vi "Plot AS Effects by Wavelength.vi"() -> ()   [LabVIEW 2019]
uses:
  <vilib>/Analysis/baseanly.llb/Mean (DBL).vi
  <vilib>/Analysis/NI_AALBase.lvlib
panel:
  in  "Color 3":u32(colorbox)=16711680
  out "New Vector - Depth":dbl[](graph)
  out "Vector - Wavelength":dbl[](graph)
  out "Vector - Abs":dbl[](graph)
  out "Vector - Scattering":dbl[](graph)
  out "Vector - Depth":dbl[](graph)
  in  "Color 1":u32(colorbox)
  in  "Color 2":u32(colorbox)=16711680
  out "WD":dbl
  in  "Array 2":T1(array[cluster])
  out "Effects by Wavelength 2":cluster{dbl[], dbl[]}[](graph)
  out "Effects by Wavelength":cluster{dbl[], dbl[]}[](graph)
  out "Graphs":T2(array[cluster])
  out "Values":dbl[][][](array[numeric])
  out "Axis Vectors":T3
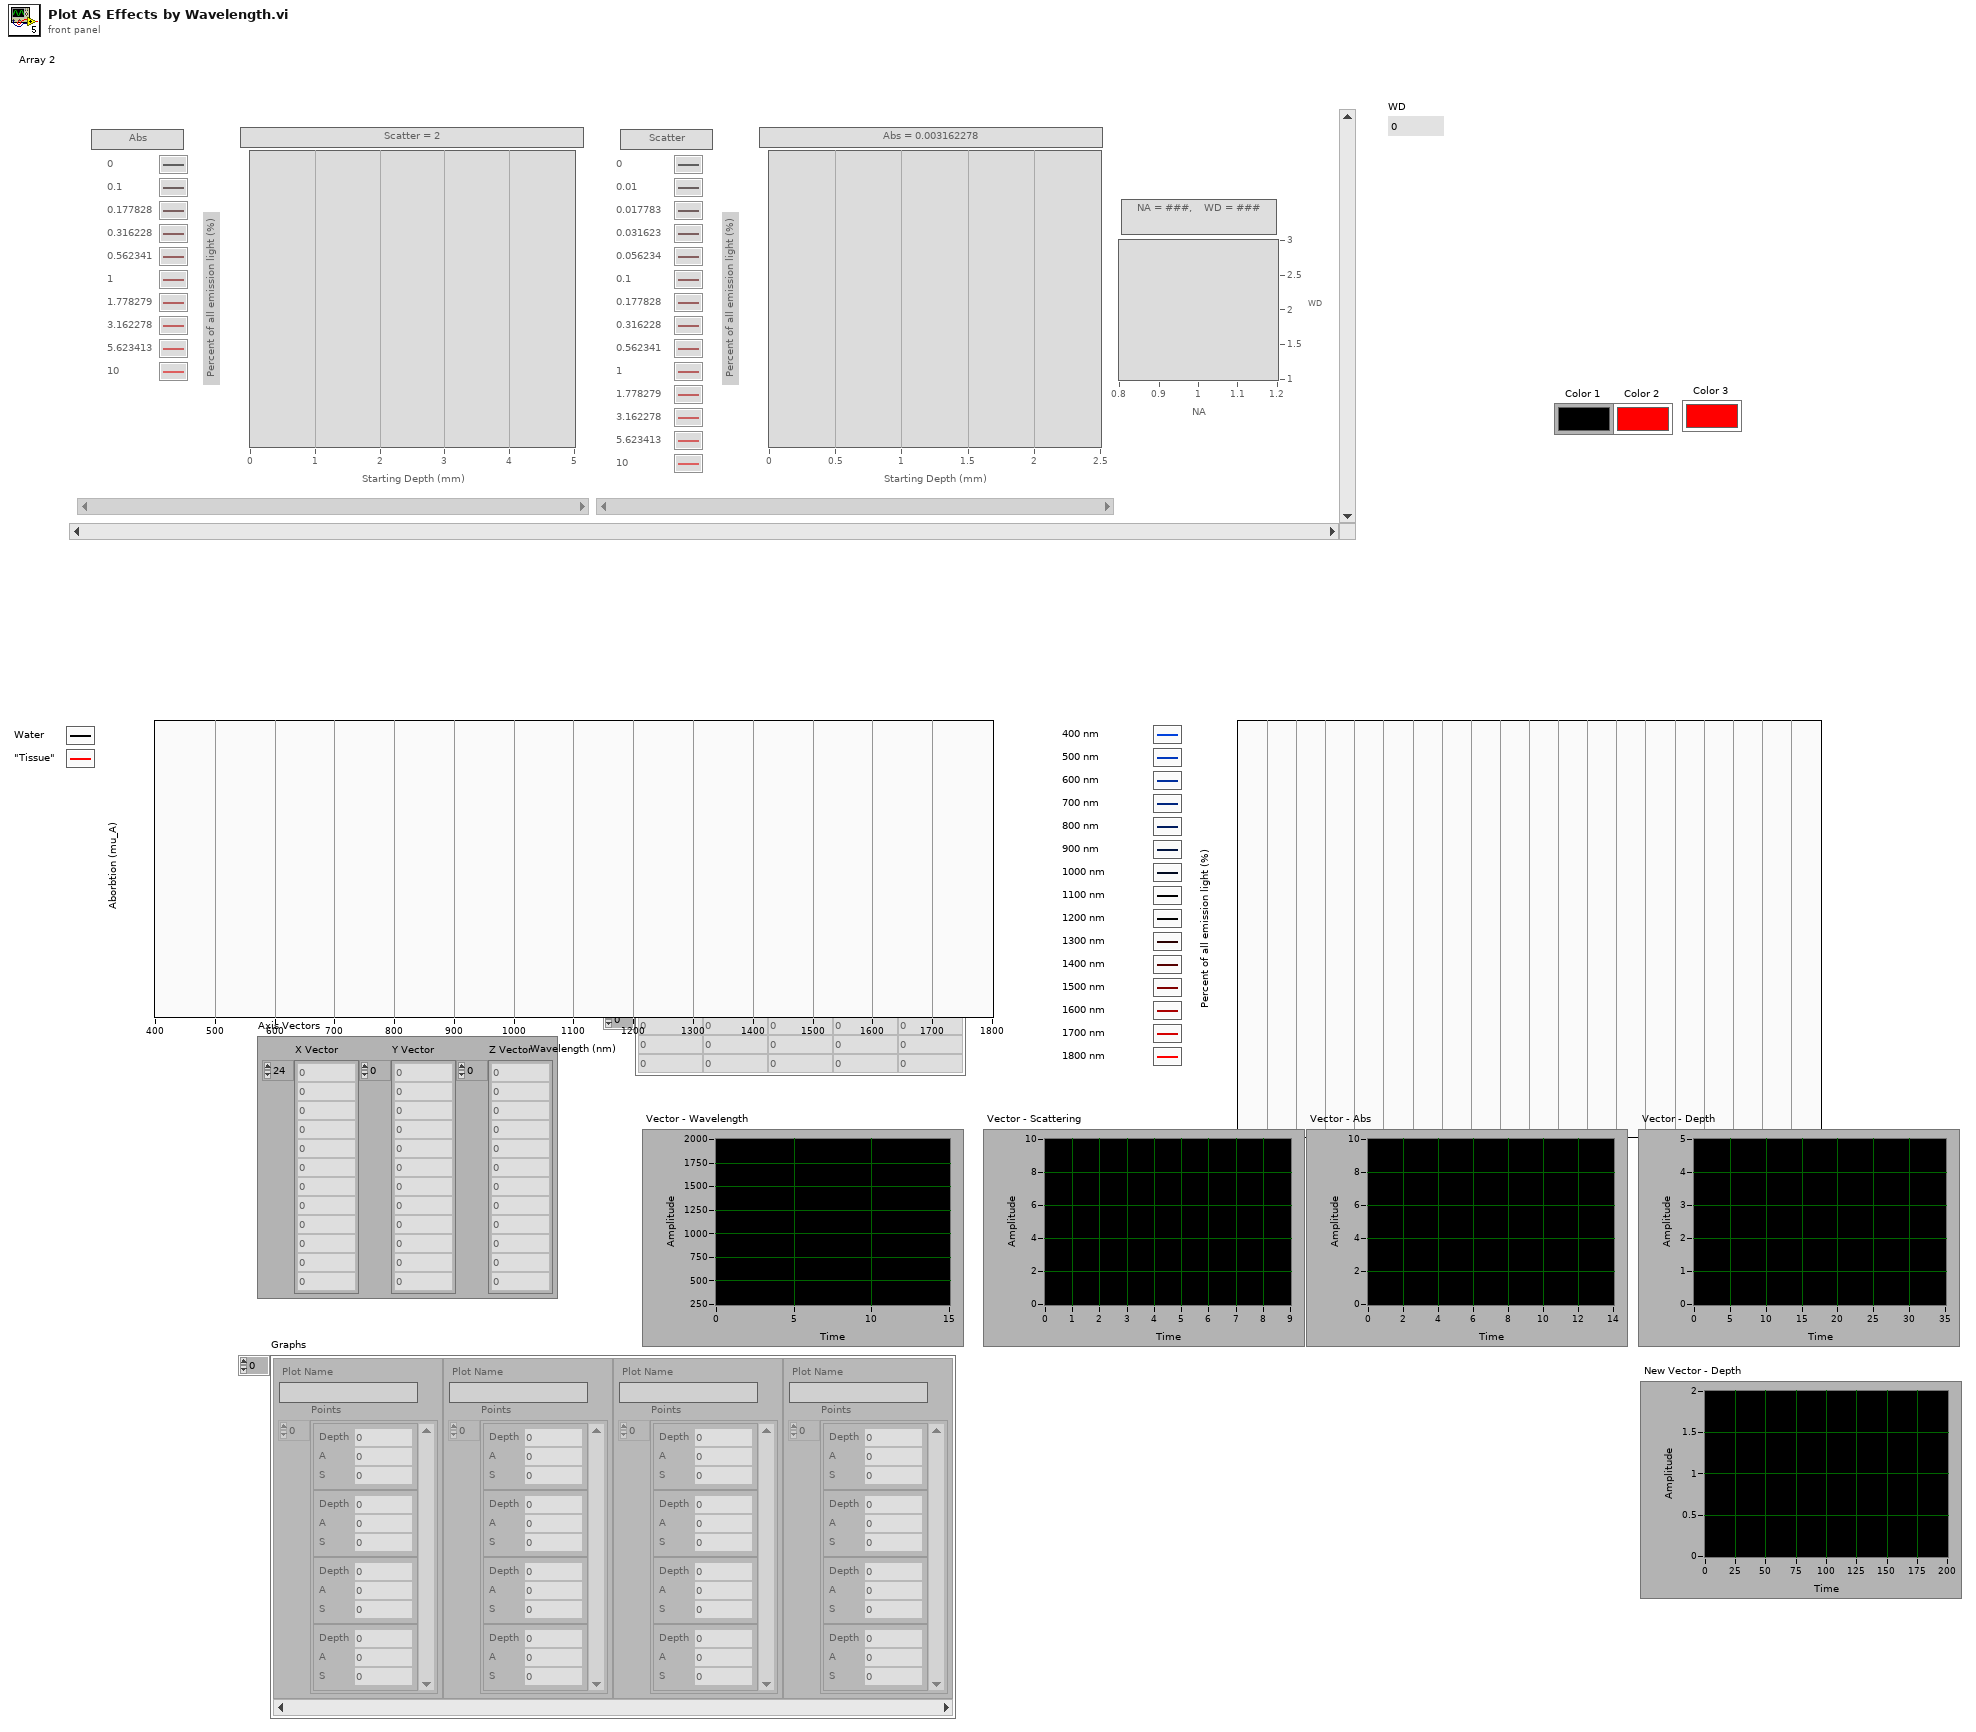
[diagram p1: front panel]
types:
  T1 = cluster{"Slab C=A, T=S 2":cluster{"Color and Time Graph":cluster{dbl[], dbl[]}[], "String":string, "String 2":string}[], "Slab C=S, T=A":cluster{"Color and Time Flipped Graph":cluster{dbl[], dbl[]}[], "String":string, "String 2":string}[], "Supra-Space Label":string, "Supra-Space Mini Map":cluster{dbl[], dbl[]}[]}[][]
  T2 = cluster{"Plot Name":string, "Points":cluster{"Depth":dbl, "A":dbl, "S":dbl}[]}[]
  T3 = cluster{"X Vector":dbl[], "Y Vector":dbl[], "Z Vector":dbl[]}
  T4 = cluster{"Slab C=A, T=S 2":cluster{"Color and Time Graph":cluster{dbl[], dbl[]}[], "String":string, "String 2":string}[], "Slab C=S, T=A":cluster{"Color and Time Flipped Graph":cluster{dbl[], dbl[]}[], "String":string, "String 2":string}[], "Supra-Space Label":string, "Supra-Space Mini Map":cluster{dbl[], dbl[]}[]}
  T5 = cluster{"Color and Time Graph":cluster{dbl[], dbl[]}[], "String":string, "String 2":string}[]
  T6 = cluster{string, cluster{dbl, "mean":dbl, "mean":dbl}[]}
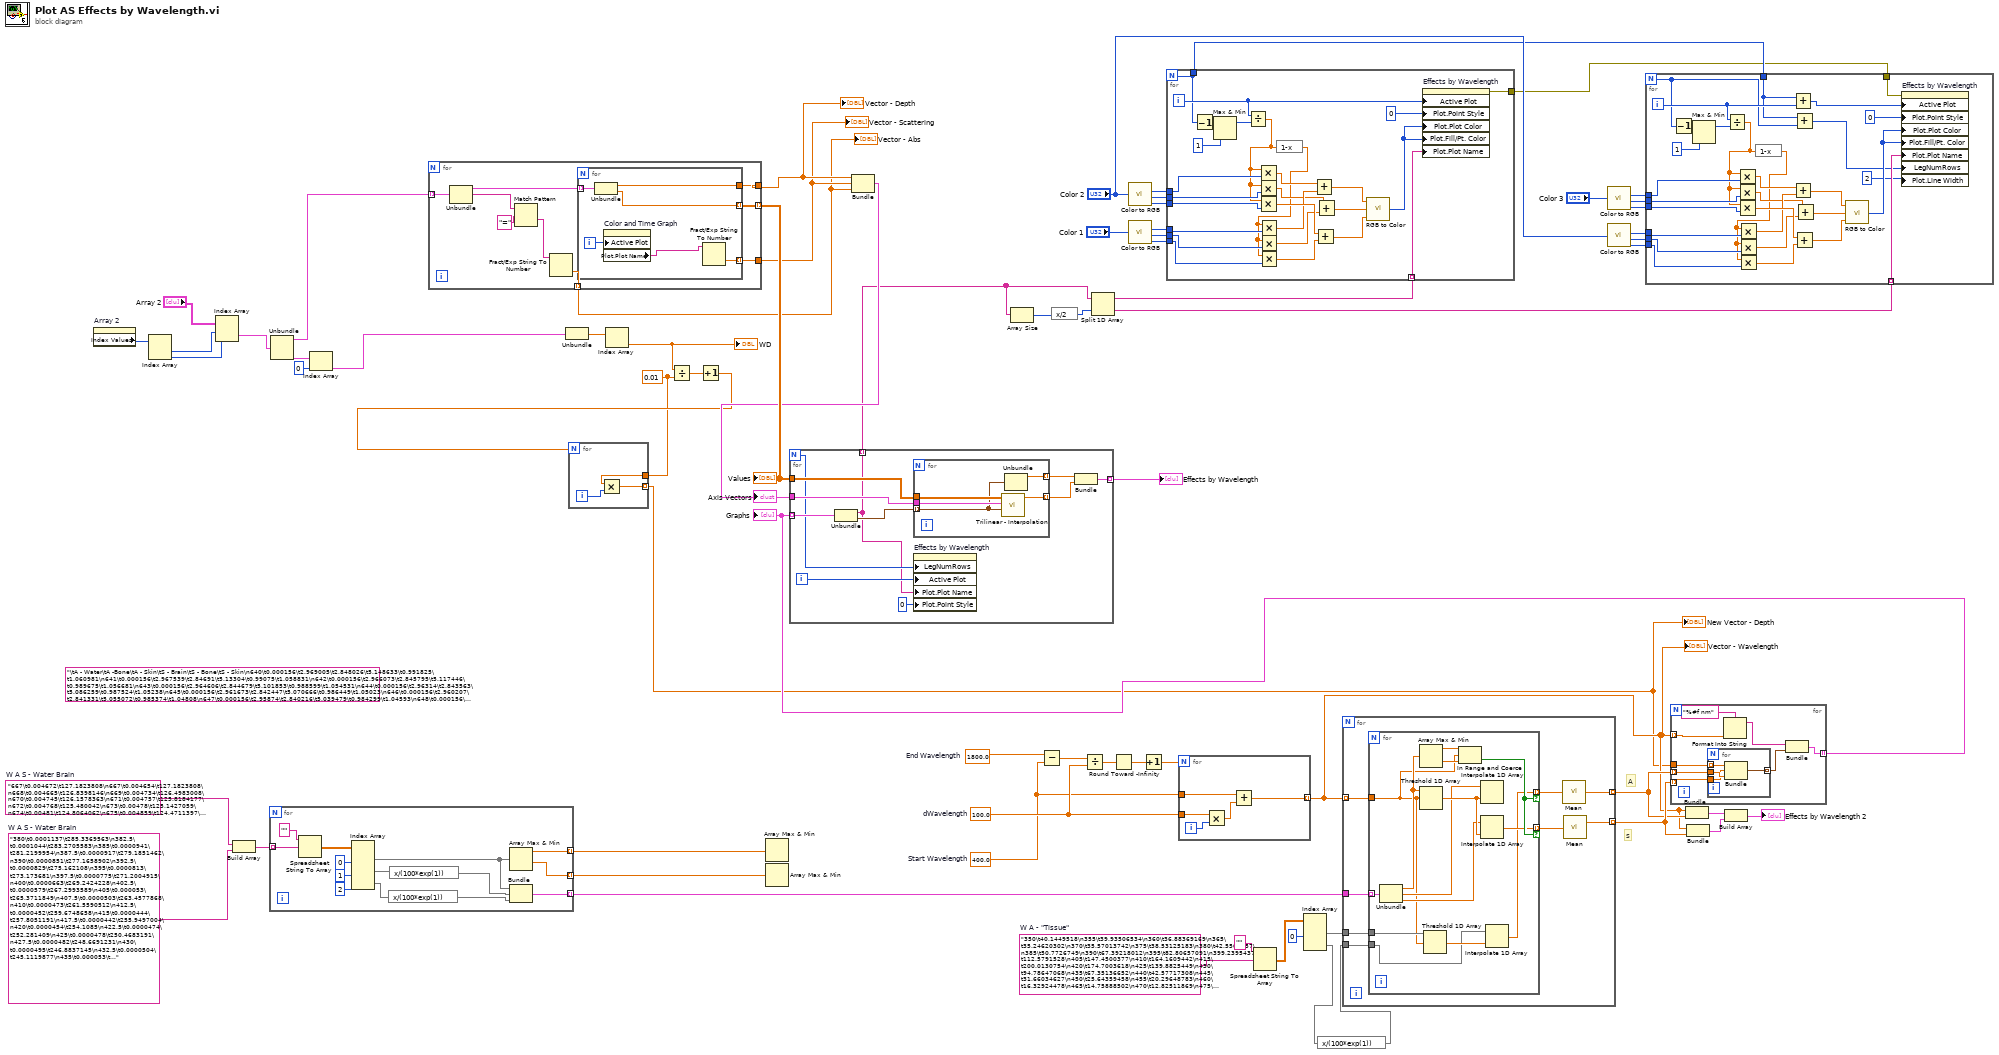
[diagram p0: block diagram]
diagram:
  w6 = "350\t40.1449518\n355\t39.93506534\n360\t36.88369169\n365\t35.24620302\n370\t35.57013742\n375\t38.53125183\n380\t42.5502257\n385\t50.7726749\n390\t67.39218012\n395\t82.80657091\n399.2395437\t112.5791528\n405\t147.4500377\n410\t164.1609442\n415\t200.0130754\n420\t174.7003618\n425\t139.8825449\n430\t94.78647068\n435\t67.35136652\n440\t42.57717308\n445\t31.66034627\n450\t25.64359458\n455\t20.29648783\n460\t16.32924478\n465\t14.75888502\n470\t12.82511869\n475\t11.17993961\n480\t10.46687393\n485\t9.635143522\n490\t9.070944487\n495\t8.526317886\n500\t7.944068527\n505\t7.865547206\n510\t7.700269633\n515\t8.291297449\n520\t10.14066835\n525\t11.9882333\n530\t15.26433309\n535\t18.44669386\n540\t20.06695237\n545\t18.73208821\n550\t16.22399299\n555\t14.2878093\n560\t12.8688612\n565\t14.58935325\n570\t17.42869783\n575\t20.36742691\n580\t18.23646398\n585\t10.31152261\n590\t5.804468682\n595\t3.200359382\n595.4372624\t2.526479178\n600\t1.325426446\n600\t1.770203167\n605\t0.905448403\n610\t0.676965894\n615\t0.503195306\n620\t0.392170144\n625\t0.332756249\n630\t0.262305095\n634.9809886\t0.217724537\n645\t0.185248241\n650\t0.170446221\n655\t0.160044101\n660\t0.149831499\n665\t0.141595627\n670\t0.138511159\n675\t0.129196263\n680\t0.125722595\n690\t0.126946584\n695\t0.124976166\n700\t0.129381074\n705\t0.132661431\n710\t0.139652936\n715\t0.14352338\n720\t0.152435705\n725\t0.161474142\n730\t0.171771141\n735\t0.18862398\n745\t0.221099782\n750\t0.22825934\n755\t0.244064738\n760\t0.256883178\n765\t0.263882999\n770\t0.280363387\n775\t0.286602175\n780\t0.295060702\n785\t0.303809506\n790\t0.307356933\n795\t0.318984637\n800\t0.318026227\n805\t0.338556011\n810\t0.34704747\n815\t0.356807245\n820\t0.375667111\n825\t0.384516469\n830\t0.398029786\n835\t0.396401541\n840\t0.417394879\n845\t0.429067561\n850\t0.437298168\n855\t0.446551299\n860\t0.451377547\n865\t0.463879395\n870\t0.470866705\n875\t0.481680183\n880\t0.491192221\n885\t0.489926302\n890\t0.501477925\n895\t0.49950668\n900\t0.510710562\n905\t0.519552579\n910\t0.524750128\n915\t0.530537466\n925\t0.573360204\n930\t0.60325251\n935\t0.652823151\n940\t0.692541\n945\t0.720914259\n950\t0.750743305\n955\t0.763756172\n960\t0.780625173\n965\t0.778987403\n970\t0.77900704\n975\t0.779424043\n980\t0.747885452\n985\t0.73604543\n990\t0.726568849\n995\t0.703054919\n1005\t0.640459172\n1010\t0.631019981\n1015\t0.605494507\n1020\t0.593542803\n1025\t0.577902355\n1030\t0.551214031\n1035\t0.52392221\n1040\t0.518082861\n1045\t0.500688926\n1050\t0.494941961\n1055\t0.490235149\n1060\t0.48120179\n1065\t0.481679295\n1070\t0.48195256\n1075\t0.485853895\n1080\t0.4910582\n1085\t0.497427334\n1090\t0.50207148\n1095\t0.508977606\n1100\t0.532046234\n1105\t0.600127102\n1110\t0.673697238\n1115\t0.737622627\n1120\t0.772759251\n1125\t0.814359969\n1130\t0.838194475\n1135\t0.869665233\n1140\t0.907133059\n1145\t0.953829503\n1150\t1.003180636\n1155\t1.029832409\n1160\t1.083120174\n1165\t1.096412814\n1170\t1.130980203\n1175\t1.166048877\n1180\t1.203815485\n1185\t1.212393847\n1190\t1.211334263\n1195\t1.202370275\n1205\t1.147063957\n1210\t1.14480334\n1215\t1.133019682\n1220\t1.123946852\n1225\t1.106075064\n1230\t1.096576616\n1235\t1.079514875\n1240\t1.071173164\n1245\t1.059883956\n1250\t1.072363897\n1255\t1.0802166\n1260\t1.078551226\n1265\t1.103983447\n1270\t1.100520936\n1275\t1.135796167\n1280\t1.14528267\n1285\t1.167016028\n1290\t1.195557654\n1295\t1.212261598\n1300\t1.2528459\n1305\t1.308400792\n1310\t1.364621761\n1315\t1.389609815\n1320\t1.4575677\n1325\t1.575745643\n1330\t1.642634392\n1335\t1.755508464\n1340\t1.848687825\n1345\t2.029670114\n1350\t2.17465122\n1355\t2.387127826\n1360\t2.725223028\n1365\t3.099532802\n1370\t3.821496699\n1375\t4.648516526\n1380\t5.387499682\n1385\t6.405116468\n1390\t7.584722337\n1395\t9.418840656\n1400\t11.03777779\n1405\t13.21466549\n1410\t13.69427731\n1415\t15.97982135\n1420\t17.72345799\n1425\t19.17000525\n1430\t20.47042995\n1435\t21.66822653\n1440\t22.35531618\n1445\t22.54541213\n1450\t22.54017823\n1455\t22.49699476\n1460\t21.75668848\n1465\t20.74741653\n1470\t19.36922072\n1475\t17.65023139\n1480\t16.86251361\n1485\t16.06846979\n1490\t15.26443185\n1495\t14.62214346\n1500\t13.84442241\n1505\t13.18146958\n1510\t12.67839918\n1515\t11.9108062\n1520\t11.18185614\n1525\t10.75134473\n1530\t10.4644584\n1535\t9.960937877\n1540\t9.500840415\n1545\t9.043900037\n1550\t8.59139503\n1555\t8.246474109\n1560\t7.787345858\n1565\t7.426642643\n1570\t7.139772584\n1575\t6.843935199\n1580\t6.471933806\n1585\t6.319686367\n1590\t5.977637406\n1595\t5.598292552\n1605\t5.088303625\n1610\t5.218338934\n1615\t5.040110752\n1620\t4.814515468\n1625\t4.683044053\n1630\t4.549824308\n1635\t4.321414117\n1640\t4.234176712\n1645\t4.146068224\n1650\t3.980268622\n1655\t3.983481534\n1660\t3.85388727\n1665\t3.845634415\n1670\t3.844005614\n1675\t3.844025551\n1680\t3.844058246\n1685\t3.843825774\n1690\t3.842531257\n1695\t3.853006003\n1700\t3.812756788\n1705\t3.993046892\n1710\t4.118971368\n1715\t4.251713554\n1720\t4.391401881\n1725\t4.600454261\n1730\t4.81775904\n1735\t5.023875653\n1740\t5.129042685\n1745\t5.3305322\n1750\t5.565698916\n1755\t5.723454663\n1760\t5.899438259\n1765\t6.09319314\n1770\t6.192110419\n1775\t6.463619324\n1780\t6.595917836\n1785\t6.588767301\n1790\t6.565100324\n1795\t6.375994569\n1805\t6.467197127\n1810\t6.978660754\n1815\t7.113147564\n1820\t7.275532454\n1825\t7.634295763\n1830\t7.706014548\n1835\t8.113183192\n1840\t8.510845753\n1845\t9.371650726\n1850\t10.0057303\n1855\t10.67490914\n1860\t12.92043247\n1865\t14.73406603\n1870\t18.52749241\n1875\t22.06098103\n1880\t26.11212325\n1885\t33.31211384\n1890\t38.47333909\n1895\t44.54571665\n1900\t54.57154096\n1905\t61.23449331\n1910\t72.21092231\n1915\t81.43598948\n1920\t88.57123236\n1925\t90.28969599\n1930\t89.89725373\n1935\t91.92493944\n1940\t91.7611798\n1945\t88.90434479\n1950\t86.04389\n1955\t83.52977617\n1960\t79.95489241\n1965\t78.8923421\n1970\t76.59635098\n1975\t72.69370288\n1985.551331\t62.41825263\n1996.197719\t53.86107465"  # W A - "Tissue"
  w24 = 1800.0  # End Wavelength
  w31 = 400.0  # Start Wavelength
  w66 = 100.0  # dWavelength
  w40 = 0.01 ("y")
  w61 = "667\t0.004672\t127.1823808\n667\t0.004654\t127.1823808\n668\t0.004665\t126.8398146\n669\t0.004734\t126.4983008\n670\t0.004745\t126.1578363\n671\t0.004757\t125.8184177\n672\t0.004768\t125.480042\n673\t0.00478\t125.1427059\n674\t0.00481\t124.8064062\n675\t0.004859\t124.4711397\n676\t0.004908\t124.1369033\n676\t0.004852\t124.1369033\n677\t0.0049\t123.8036937\n678\t0.00493\t123.4715078\n679\t0.004978\t123.1403426\n680\t0.005008\t122.8101948\n681\t0.005038\t122.4810613\n682\t0.00503\t122.152939\n683\t0.005078\t121.8258247\n684\t0.005126\t121.4997155\n685\t0.005173\t121.1746082\n686\t0.005202\t120.8504998\n687\t0.00525\t120.5273871\n688\t0.005315\t120.2052671\n689\t0.005362\t119.8841368\n689.7\t0.00543\t119.6599327\n690\t0.005536\t119.563993\n691\t0.005638\t119.2448329\n692\t0.00572\t118.9266533\n693\t0.005803\t118.6094513\n694\t0.005921\t118.2932238\n695\t0.006021\t117.9779679\n696\t0.006139\t117.6636805\n697\t0.006256\t117.3503587\n698\t0.006391\t117.0379995\n699\t0.006526\t116.7266001\n700\t0.006678\t116.4161573\n701\t0.00683\t116.1066683\n702\t0.006981\t115.7981301\n703\t0.00715\t115.4905399\n704\t0.007354\t115.1838947\n705\t0.007522\t114.8781916\n706\t0.007725\t114.5734278\n707\t0.007927\t114.2696002\n708\t0.008147\t113.9667061\n709\t0.008401\t113.6647426\n710\t0.008655\t113.3637068\n711\t0.008979\t113.0635959\n712\t0.009301\t112.7644071\n713\t0.009694\t112.4661374\n714\t0.010067\t112.1687841\n715\t0.010492\t111.8723444\n716\t0.010952\t111.5768154\n717\t0.01141\t111.2821944\n718\t0.011901\t110.9884786\n719\t0.012427\t110.6956652\n721\t0.01295\t110.1127344\n722\t0.013489\t109.8226115\n723\t0.014061\t109.5333799\n724\t0.014667\t109.245037\n725\t0.015253\t108.95758\n726\t0.015924\t108.6710061\n727\t0.016646\t108.3853127\n728\t0.017607\t108.100497\n729\t0.018444\t107.8165563\n730\t0.019624\t107.533488\n731\t0.020801\t107.2512894\n732\t0.021974\t106.9699578\n733\t0.023144\t106.6894905\n734\t0.024482\t106.4098849\n735\t0.025304\t106.1311383\n736\t0.026123\t105.8532482\n738\t0.026733\t105.3000265\n739\t0.027377\t105.0246898\n740\t0.02768\t104.750199\n741\t0.027982\t104.4765515\n742\t0.028113\t104.2037448\n743\t0.028245\t103.9317762\n744\t0.028376\t103.6606432\n745\t0.028338\t103.3903432\n746\t0.028468\t103.1208736\n747\t0.02843\t102.8522319\n748\t0.02856\t102.5844156\n750\t0.028484\t102.0512489\n751\t0.028613\t101.7858934\n752\t0.028575\t101.5213533\n753\t0.028704\t101.2576258\n754\t0.028666\t100.9947086\n755\t0.028794\t100.7325992\n756\t0.028756\t100.4712951\n758\t0.028681\t99.95109276\n759\t0.028643\t99.69218966\n760\t0.028605\t99.43408199\n761\t0.028733\t99.1767673\n762\t0.028695\t98.92024318\n763\t0.028657\t98.66450717\n765\t0.028582\t98.15538985\n766\t0.028545\t97.90200372\n767\t0.028344\t97.64939606\n768\t0.028307\t97.3975645\n769\t0.02827\t97.14650665\n770\t0.028234\t96.89622012\n772\t0.027998\t96.39795159\n773\t0.027799\t96.14996486\n774\t0.027763\t95.90274003\n775\t0.027565\t95.65627475\n776\t0.027529\t95.41056669\n778\t0.027297\t94.92141292\n779\t0.027101\t94.67796259\n780\t0.026905\t94.43526021\n781\t0.026549\t94.1933035\n783\t0.02632\t93.71161788\n784\t0.026127\t93.47188442\n785\t0.025933\t93.2328875\n786\t0.02558\t92.99462485\n787\t0.025229\t92.75709422\n789\t0.025005\t92.28422003\n790\t0.024656\t92.04887198\n791\t0.024465\t91.81424701\n792\t0.024117\t91.58034287\n794\t0.02374\t91.11468828\n795\t0.023552\t90.88293341\n796\t0.023365\t90.65189056\n797\t0.023178\t90.42155755\n799\t0.022805\t89.96301233\n800\t0.022462\t89.73479577\n801\t0.022434\t89.50728037\n803\t0.022222\t89.05434442\n804\t0.022038\t88.82891958\n805\t0.022011\t88.60418731\n807\t0.021956\t88.15679201\n808\t0.021773\t87.93412473\n809\t0.021902\t87.71214156\n810\t0.021875\t87.49084039\n812\t0.021976\t87.05027569\n813\t0.022103\t86.83100798\n814\t0.02223\t86.61241393\n816\t0.022484\t86.17723855\n817\t0.022764\t85.96065309\n818\t0.023043\t85.74473304\n820\t0.023294\t85.31488105\n821\t0.023878\t85.10094502\n822\t0.02446\t84.88766628\n824\t0.025163\t84.46307255\n825\t0.026199\t84.25175355\n826\t0.027689\t84.04108379\n828\t0.029139\t83.62168401\n829\t0.031075\t83.41295003\n831\t0.032966\t82.99740397\n832\t0.034588\t82.79058797\n833\t0.036055\t82.58440737\n835\t0.037022\t82.17394459\n836\t0.037879\t81.96965851\n838\t0.038539\t81.56296733\n839\t0.039092\t81.36055837\n840\t0.039494\t81.15877128\n842\t0.039997\t80.75705505\n843\t0.040397\t80.55712211\n845\t0.040748\t80.15909711\n846\t0.041145\t79.96100129\n848\t0.041493\t79.56663361\n849\t0.042036\t79.37035802\n850\t0.041986\t79.17468545\n851\t0.042232\t78.97961405\n853\t0.042723\t78.59126737\n855\t0.043064\t78.20530328\n856\t0.043601\t78.01321013\n858\t0.043792\t77.63079252\n859\t0.044326\t77.44046445\n861\t0.044661\t77.06156075\n862\t0.045047\t76.87298154\n864\t0.045524\t76.49755946\n865\t0.046052\t76.31071304\n866\t0.04658\t76.12444067\n868\t0.047052\t75.75361104\n870\t0.047521\t75.38505651\n871\t0.048332\t75.20162805\n873\t0.048941\t74.83646005\n874\t0.049604\t74.65471706\n876\t0.050495\t74.29290446\n877\t0.051154\t74.11283144\n879\t0.052038\t73.75434342\n880\t0.052979\t73.57592502\n882\t0.053856\t73.22073103\n883\t0.054649\t73.04395206\n885\t0.055661\t72.69202182\n887\t0.056527\t72.34225074\n888\t0.057454\t72.16817074\n890\t0.058314\t71.82161359\n891\t0.059235\t71.64913316\n893\t0.060088\t71.3057604\n895\t0.060936\t70.96449431\n896\t0.06185\t70.79464721\n898\t0.062692\t70.4565169\n899\t0.063601\t70.28823047\n901\t0.064575\t69.95320712\n902\t0.065618\t69.78646702\n904\t0.066724\t69.45452208\n906\t0.067686\t69.12461369\n907\t0.068997\t68.9604193\n909\t0.070366\t68.63354232\n911\t0.071867\t68.30867081\n912\t0.073579\t68.14698324\n914\t0.075618\t67.82509686\n916\t0.077922\t67.50518531\n917\t0.080852\t67.34596631\n919\t0.084095\t67.02899432\n921\t0.088006\t66.71396701\n922\t0.09268\t66.55717888\n924\t0.098192\t66.24504626\n926\t0.104222\t65.93482863\n928\t0.11131\t65.62651424\n929\t0.119441\t65.47306711\n931\t0.128093\t65.16758572\n933\t0.137382\t64.86397852\n935\t0.146496\t64.56223401\n936\t0.155737\t64.41205668\n938\t0.168802\t64.1130848\n940\t0.181811\t63.81594716\n941\t0.196308\t63.66806267\n943\t0.21055\t63.37365533\n945\t0.228721\t63.08105424\n947\t0.246816\t62.79024831\n949\t0.270131\t62.50122654\n950\t0.297625\t62.35738128\n952\t0.327359\t62.07101523\n954\t0.362238\t61.78640609\n956\t0.393028\t61.50354308\n958\t0.418442\t61.22241549\n960\t0.438514\t60.94301267\n961\t0.453749\t60.80395475\n963\t0.463246\t60.52711927\n965\t0.470099\t60.25198223\n967\t0.475625\t59.97853321\n969\t0.478534\t59.70676185\n971\t0.48143\t59.43665786\n973\t0.484315\t59.16821101\n974\t0.486399\t59.03460584\n976\t0.486689\t58.76862566\n978\t0.485694\t58.50427732\n980\t0.482138\t58.2415508\n982\t0.478597\t57.98043617\n984\t0.473793\t57.72092353\n986\t0.467734\t57.46300304\n988\t0.460428\t57.20666495\n990\t0.453151\t56.95189954\n992\t0.44337\t56.69869717\n994\t0.436157\t56.44704824\n996\t0.426449\t56.19694323\n998\t0.41678\t55.94837266\n1000\t0.40715\t55.70132712\n1002\t0.396305\t55.45579725\n1004\t0.386754\t55.21177376\n1006\t0.375992\t54.9692474\n1008\t0.364026\t54.72820898\n1010\t0.352107\t54.48864938\n1012\t0.340236\t54.25055952\n1014\t0.32965\t54.0139304\n1016\t0.319107\t53.77875304\n1018\t0.308604\t53.54501853\n1020\t0.295679\t53.31271804\n1022\t0.284034\t53.08184275\n1024\t0.272435\t52.85238393\n1026\t0.262106\t52.62433288\n1028\t0.250594\t52.39768097\n1030\t0.239127\t52.17241961\n1033\t0.229917\t51.83711621\n1035\t0.21976\t51.61529403\n1037\t0.210853\t51.39483277\n1039\t0.201981\t51.17572408\n1041\t0.19435\t50.95795966\n1043\t0.186749\t50.74153128\n1046\t0.179005\t50.41937583\n1048\t0.171469\t50.20625176\n1050\t0.166355\t49.99443524\n1052\t0.16126\t49.78391826\n1054\t0.156185\t49.57469285\n1057\t0.152176\t49.26325908\n1059\t0.149515\t49.05722801\n1061\t0.14568\t48.85246098\n1063\t0.144224\t48.64895024\n1066\t0.142639\t48.34602281\n1068\t0.141195\t48.14561916\n1070\t0.140931\t47.94644503\n1073\t0.140537\t47.64997268\n1075\t0.141445\t47.45383944\n1077\t0.143516\t47.25890951\n1080\t0.144281\t46.96875469\n1082\t0.147498\t46.77680085\n1084\t0.151863\t46.58602469\n1087\t0.156068\t46.30205278\n1089\t0.160397\t46.11418929\n1091\t0.165862\t45.92747837\n1094\t0.171151\t45.64955762\n1096\t0.177718\t45.46569731\n1098\t0.18655\t45.28296502\n1101\t0.19289\t45.01096649\n1103\t0.200515\t44.83102406\n1106\t0.207925\t44.56317826\n1108\t0.216622\t44.3859831\n1111\t0.225086\t44.12222664\n1113\t0.233714\t43.9477368\n1116\t0.235338\t43.68800723\n1118\t0.245033\t43.51618141\n1121\t0.257829\t43.26041726\n1123\t0.271917\t43.09121479\n1126\t0.289049\t42.83935551\n1128\t0.316387\t42.67273633\n1131\t0.353325\t42.42472231\n1133\t0.403721\t42.26064699\n1136\t0.471239\t42.01641952\n1139\t0.557157\t41.77443617\n1141\t0.651997\t41.61435048\n1144\t0.753543\t41.37606161\n1146\t0.859689\t41.21842002\n1149\t0.949313\t40.98376922\n1152\t1.040653\t40.75127455\n1154\t1.09983\t40.59746616\n1157\t1.140423\t40.36852109\n1160\t1.169972\t40.14167972\n1162\t1.189588\t39.99161131\n1165\t1.197311\t39.76823324\n1168\t1.204994\t39.54690771\n1171\t1.212639\t39.32761587\n1173\t1.231997\t39.1825419\n1176\t1.228854\t38.96659809\n1179\t1.236386\t38.75263852\n1182\t1.243879\t38.54064495\n1184\t1.252392\t38.4003992\n1187\t1.259813\t38.19164224\n1190\t1.267197\t37.98480347\n1193\t1.274544\t37.77986528\n1196\t1.281854\t37.57681019\n1199\t1.278646\t37.37562091\n1201\t1.266054\t37.24252281\n1204\t1.273336\t37.04440518\n1207\t1.25976\t36.84810799\n1210\t1.256637\t36.65361451\n1213\t1.243169\t36.46090816\n1216\t1.240102\t36.26997252\n1219\t1.216433\t36.08079133\n1222\t1.213447\t35.89334846\n1225\t1.200217\t35.70762794\n1228\t1.197284\t35.52361394\n1231\t1.184158\t35.34129078\n1234\t1.171096\t35.16064293\n1237\t1.158097\t34.981655\n1240\t1.155295\t34.80431172\n1243\t1.142397\t34.62859799\n1246\t1.129561\t34.45449883\n1250\t1.115894\t34.22485256\n1253\t1.103193\t34.05446328\n1256\t1.100558\t33.88563965\n1259\t1.097935\t33.71836729\n1262\t1.085368\t33.55263193\n1265\t1.082794\t33.38841946\n1269\t1.079381\t33.17181427\n1272\t1.086714\t33.011101\n1275\t1.103869\t32.85186448\n1278\t1.111111\t32.69409112\n1282\t1.137051\t32.48597947\n1285\t1.163734\t32.33156811\n1288\t1.180536\t32.17857559\n1292\t1.215787\t31.97677011\n1295\t1.251785\t31.8270377\n1298\t1.297299\t31.67868113\n1302\t1.351223\t31.48299074\n1305\t1.415522\t31.3377955\n1308\t1.489134\t31.19393441\n1312\t1.580374\t31.0041738\n1315\t1.672331\t30.86337825\n1319\t1.791113\t30.67766125\n1322\t1.910621\t30.53986591\n1326\t2.04701\t30.35810636\n1329\t2.203133\t30.2232473\n1333\t2.356784\t30.04536086\n1336\t2.539611\t29.91337552\n1340\t2.700832\t29.73927966\n1344\t2.889143\t29.56731348\n1347\t3.097279\t29.43972075\n1351\t3.236933\t29.27141899\n1355\t3.394311\t29.10517603\n1358\t3.553377\t28.98182973\n1362\t3.72747\t28.81912923\n1366\t3.955739\t28.65841902\n1369\t4.222447\t28.53917781\n1373\t4.640313\t28.38189217\n1377\t5.183514\t28.22653056\n1381\t5.987452\t28.07306945\n1385\t7.204114\t27.9214856\n1388\t8.781973\t27.80901582\n1392\t11.013629\t27.66066207\n1396\t13.952631\t27.51412309\n1400\t16.964599\t27.36937668\n1404\t19.690893\t27.22640092\n1408\t22.312447\t27.08517414\n1412\t24.652156\t26.94567496\n1416\t26.357429\t26.80788224\n1420\t27.699111\t26.6717751\n1424\t29.121504\t26.53733292\n1428\t30.271928\t26.40453534\n1432\t31.064909\t26.27336224\n1437\t32.006203\t26.11165004\n1440\t32.201323\t26.01581023\n1445\t32.524722\t25.8580302\n1449\t32.69511\t25.73354236\n1453\t32.778075\t25.61057735\n1457\t32.688087\t25.48911654\n1462\t32.404388\t25.33937779\n1466\t31.544503\t25.22123449\n1470\t30.603813\t25.10453641\n1474\t29.668228\t24.98926587\n1479\t28.208484\t24.84715859\n1484\t26.927936\t24.70722093\n1488\t25.75768\t24.59681064\n1492\t24.08835\t24.48775098\n1497\t22.916627\t24.35330057\n1501\t21.599757\t24.24721971\n1506\t20.443298\t24.1164416\n1510\t19.224049\t24.01325817\n1515\t18.082301\t23.88605207\n1519\t17.04195\t23.78568694\n1524\t16.079017\t23.66195527\n1529\t15.368942\t23.54011268\n1533\t14.591088\t23.44397934\n1538\t13.8083\t23.32546469\n1543\t12.786261\t23.20875946\n1548\t12.176715\t23.09383602\n1552\t11.659519\t23.00316187\n1557\t10.976405\t22.89137739\n1562\t10.458567\t22.78129958\n1567\t9.944032\t22.67290238\n1572\t9.51271\t22.56616013\n1577\t9.163808\t22.46104757\n1582\t8.817112\t22.35753981\n1587\t8.4726\t22.25561236\n1592\t8.130252\t22.15524108\n1597\t7.868735\t22.05640222\n1602\t7.608851\t21.95907237\n1607\t7.381863\t21.86322851\n1612\t7.19526\t21.76884795\n1618\t6.989946\t21.65749138\n1623\t6.805816\t21.5662519\n1628\t6.661411\t21.47640542\n1634\t6.49083\t21.37039848\n1640\t6.356022\t21.26633071\n1644\t6.267897\t21.19801197\n1650\t6.161329\t21.09709765\n1655\t6.051599\t21.01441397\n1661\t5.984346\t20.91685818\n1666\t5.921129\t20.83692631\n1672\t5.877333\t20.74261729\n1677\t5.83733\t20.66534563\n1683\t5.838919\t20.57417532\n1689\t5.833057\t20.48467277\n1690\t5.852931\t20.46991567\n1700\t5.89141\t20.32481547\n1706\t5.922252\t20.23987444\n1710\t6.011599\t20.18411208\n1718\t6.136894\t20.0746254\n1724\t6.275896\t19.99426107\n1730\t6.442989\t19.91536683\n1740\t6.652358\t19.78707049\n1742\t6.917996\t19.76188156\n1748\t7.260889\t19.68723822\n1754\t7.594271\t19.61396032\n1760\t7.925381\t19.54202288\n1770\t8.396555\t19.42503956\n1773\t8.717786\t19.39064076\n1779\t8.970933\t19.32278848\n1785\t9.151978\t19.25617742\n1792\t9.186353\t19.180003\n1798\t9.155698\t19.1160039\n1805\t9.259431\t19.04281644\n1810\t9.159364\t18.99149646\n1818\t9.193219\t18.91100925\n1824\t9.231873\t18.85193082\n1831\t9.402472\t18.7843705\n1838\t9.708512\t18.71824982\n1845\t10.08034\t18.6535381\n1851\t11.133899\t18.59916956\n1860\t12.782798\t18.51947585\n1865\t15.76692\t18.47614597\n1872\t21.548102\t18.41659325\n1879\t31.767034\t18.35830953\n1890\t48.680532\t18.26921992\n1894\t72.983142\t18.23756408\n1901\t98.494957\t18.1830953\n1908\t117.233431\t18.12978719\n1920\t128.616633\t18.04103125\n1923\t134.61634\t18.01934963\n1930\t136.732523\t17.96953078\n1940\t135.010587\t17.90019692\n1945\t130.509344\t17.86632186\n1953\t123.54035\t17.81319423\n1960\t115.405439\t17.76776835\n1968\t107.27389\t17.71703713\n1976\t99.208184\t17.66753949\n1984\t91.207524\t17.61924542\n1992\t83.901968\t17.57212567\n2000\t77.283175\t17.52615167\n2008\t70.717122\t17.48129557\n2016\t65.449844\t17.43753019\n2024\t60.162117\t17.39482899\n2032\t55.410765\t17.35316612\n2040\t51.189478\t17.31251631\n2050\t47.652853\t17.2630912\n2057\t43.98535\t17.22938747\n2066\t40.448384\t17.18710726\n2074\t37.565812\t17.15049531\n2083\t34.990373\t17.11036992\n2092\t32.617299\t17.07134049\n2100\t28.723131\t17.03754351\n2100\t30.458487\t17.03754351\n2118\t26.936412\t16.96447463\n2127\t25.52267\t16.92943011\n2136\t24.297335\t16.89534277\n2145\t23.199452\t16.86218647\n2155\t22.333734\t16.8264072\n2164\t21.660148\t16.79513378\n2173\t21.049971\t16.76471454\n2183\t20.665721\t16.73188885\n2193\t20.284975\t16.70005784\n2202\t20.144998\t16.67223546\n2212\t20.053927\t16.64221206\n2222\t20.133338\t16.61309842\n2232\t20.380941\t16.58486699\n2242\t20.738434\t16.55749102\n2252\t21.204354\t16.53094459\n2262\t21.943926\t16.50520257\n2272\t22.787608\t16.48024058\n2283\t23.888763\t16.45365514\n2293\t25.209464\t16.43025513\n2304\t26.670811\t16.40533326\n2314\t28.456257\t16.38339749\n2325\t30.483581\t16.36003509\n2336\t32.653196\t16.33745022\n2347\t36.14103\t16.315617\n2358\t37.890963\t16.29451041\n2369\t40.844681\t16.27410627\n2381\t44.069378\t16.2526209\n2392\t47.544167\t16.23361089\n2403\t51.457795\t16.21523355\n2415\t55.677084\t16.19588238\n2427\t60.579534\t16.17723272\n2439\t65.433743\t16.15925913\n2451\t71.778531\t16.1419371\n2463\t79.592112\t16.12524301\n2475\t86.822193\t16.10915411\n2487\t94.487784\t16.09364844\n2500\t100.53096\t16.07748431\n"  # W A S - Water Brain
  w62 = "380\t0.0001137\t285.3369563\n382.5\t0.0001044\t283.2705583\n385\t0.0000941\t281.2199954\n387.5\t0.0000917\t279.1851462\n390\t0.0000851\t277.1658902\n392.5\t0.0000829\t275.162108\n395\t0.0000813\t273.173681\n397.5\t0.0000775\t271.2004915\n400\t0.0000663\t269.2424228\n402.5\t0.0000579\t267.2993589\n405\t0.000053\t265.3711849\n407.5\t0.0000503\t263.4577868\n410\t0.0000473\t261.5590512\n412.5\t0.0000452\t259.6748658\n415\t0.0000444\t257.8051191\n417.5\t0.0000442\t255.9497004\n420\t0.0000454\t254.1085\n422.5\t0.0000474\t252.281409\n425\t0.0000478\t250.4683191\n427.5\t0.0000482\t248.6691231\n430\t0.0000495\t246.8837145\n432.5\t0.0000504\t245.1119877\n435\t0.000053\t243.3538379\n437.5\t0.000058\t241.6091609\n440\t0.0000635\t239.8778535\n442.5\t0.0000696\t238.1598134\n445\t0.0000751\t236.4549387\n447.5\t0.000083\t234.7631287\n450\t0.0000922\t233.0842832\n452.5\t0.0000969\t231.4183028\n455\t0.0000962\t229.7650891\n457.5\t0.0000957\t228.1245441\n460\t0.0000979\t226.4965707\n462.5\t0.0001005\t224.8810727\n465\t0.0001011\t223.2779544\n467.5\t0.000102\t221.6871209\n470\t0.000106\t220.1084782\n472.5\t0.000109\t218.5419328\n475\t0.000114\t216.987392\n477.5\t0.000121\t215.4447638\n480\t0.000127\t213.9139569\n482.5\t0.000131\t212.3948807\n485\t0.000136\t210.8874453\n487.5\t0.000144\t209.3915616\n490\t0.00015\t207.9071411\n492.5\t0.000162\t206.4340957\n495\t0.000173\t204.9723385\n497.5\t0.000191\t203.5217829\n500\t0.000204\t202.082343\n502.5\t0.000228\t200.6539337\n505\t0.000256\t199.2364704\n507.5\t0.00028\t197.8298693\n510\t0.000325\t196.4340472\n512.5\t0.000372\t195.0489213\n515\t0.000396\t193.6744099\n517.5\t0.000399\t192.3104314\n520\t0.000409\t190.9569053\n522.5\t0.000416\t189.6137513\n525\t0.000417\t188.2808901\n527.5\t0.000428\t186.9582428\n530\t0.000434\t185.645731\n532.5\t0.000447\t184.3432771\n535\t0.000452\t183.0508041\n537.5\t0.000466\t181.7682354\n540\t0.000474\t180.4954952\n542.5\t0.000489\t179.2325081\n545\t0.000511\t177.9791995\n547.5\t0.000537\t176.735495\n550\t0.000565\t175.5013212\n552.5\t0.000593\t174.276605\n555\t0.000596\t173.0612739\n557.5\t0.000606\t171.855256\n560\t0.000619\t170.65848\n562.5\t0.00064\t169.4708749\n565\t0.000642\t168.2923707\n567.5\t0.000672\t167.1228974\n570\t0.000695\t165.9623859\n572.5\t0.000733\t164.8107675\n575\t0.000772\t163.6679741\n577.5\t0.000836\t162.533938\n580\t0.000896\t161.4085922\n582.5\t0.000989\t160.29187\n585\t0.0011\t159.1837054\n587.5\t0.00122\t158.0840327\n590\t0.001351\t156.992787\n592.5\t0.001516\t155.9099035\n595\t0.001672\t154.8353184\n597.5\t0.001925\t153.7689679\n600\t0.002224\t152.7107889\n602.5\t0.00247\t151.6607189\n605\t0.002577\t150.6186956\n607.5\t0.002629\t149.5846575\n610\t0.002644\t148.5585433\n612.5\t0.002665\t147.5402924\n615\t0.002678\t146.5298444\n617.5\t0.002707\t145.5271396\n620\t0.002755\t144.5321186\n622.5\t0.00281\t143.5447225\n625\t0.002834\t142.564893\n627.5\t0.002904\t141.592572\n630\t0.002916\t140.627702\n632.5\t0.002995\t139.6702259\n635\t0.003012\t138.7200871\n637.5\t0.003077\t137.7772292\n640\t0.003108\t136.8415966\n642.5\t0.00322\t135.9131338\n645\t0.00325\t134.9917859\n647.5\t0.00335\t134.0774984\n650\t0.0034\t133.1702172\n652.5\t0.00358\t132.2698885\n655\t0.00371\t131.3764592\n657.5\t0.00393\t130.4898763\n660\t0.0041\t129.6100874\n662.5\t0.00424\t128.7370404\n665\t0.00429\t127.8706837\n667.5\t0.00436\t127.0109659\n670\t0.00439\t126.1578363\n672.5\t0.00448\t125.3112442\n675\t0.00448\t124.4711397\n677.5\t0.00461\t123.637473\n680\t0.00465\t122.8101948\n682.5\t0.00478\t121.989256\n685\t0.00486\t121.1746082\n687.5\t0.00502\t120.3662032\n690\t0.00516\t119.563993\n692.5\t0.00538\t118.7679303\n695\t0.00559\t117.9779679\n697.5\t0.00592\t117.194059\n700\t0.00624\t116.4161573\n702.5\t0.00663\t115.6442167\n705\t0.00704\t114.8781916\n707.5\t0.00756\t114.1180367\n710\t0.00827\t113.3637068\n712.5\t0.00914\t112.6151575\n715\t0.01007\t111.8723444\n717.5\t0.01119\t111.1352236\n720\t0.01231\t110.4037513\n722.5\t0.01356\t109.6778845\n725\t0.01489\t108.95758\n727.5\t0.01678\t108.2427953\n"  # W A S - Water Brain
  (unwired) "\tA - Water\tA -Bone\tA - Skin\tS - Brain\tS - Bone\tS - Skin\n640\t0.000156\t2.969005\t2.848026\t5.148633\t0.991825\t1.060981\n641\t0.000156\t2.967539\t2.84691\t5.13304\t0.99075\t1.058831\n642\t0.000156\t2.966073\t2.845795\t5.117446\t0.989675\t1.056681\n643\t0.000156\t2.964606\t2.844679\t5.101853\t0.988599\t1.054531\n644\t0.000156\t2.96314\t2.843563\t5.086259\t0.987524\t1.05238\n645\t0.000156\t2.961673\t2.842447\t5.070666\t0.986449\t1.05023\n646\t0.000156\t2.960207\t2.841331\t5.055072\t0.985374\t1.04808\n647\t0.000156\t2.95874\t2.840216\t5.039479\t0.984299\t1.04593\n648\t0.000156\t2.957274\t2.8391\t5.023885\t0.983224\t1.043779\n649\t0.000156\t2.955807\t2.837984\t5.008292\t0.982149\t1.041629\n650\t0.000156\t2.954341\t2.836868\t4.992698\t0.981074\t1.039479\n651\t0.000156\t2.952874\t2.835752\t4.977154\t0.979999\t1.037499\n652\t0.000156\t2.951408\t2.834637\t4.961703\t0.978924\t1.035841\n653\t0.000156\t2.949987\t2.833525\t4.946252\t0.977848\t1.034182\n654\t0.000156\t2.948638\t2.83242\t4.930801\t0.976773\t1.032524\n655\t0.000156\t2.947288\t2.831315\t4.915349\t0.975698\t1.030865\n656\t0.000156\t2.945939\t2.83021\t4.899898\t0.974623\t1.029207\n657\t0.000156\t2.944589\t2.829104\t4.884447\t0.973589\t1.027549\n658\t0.000156\t2.94324\t2.827999\t4.868996\t0.972977\t1.02589\n659\t0.000156\t2.94189\t2.826894\t4.853545\t0.972366\t1.024232\n660\t0.000156\t2.94054\t2.825789\t4.838094\t0.971754\t1.022573\n661\t0.000156\t2.939191\t2.824684\t4.822557\t0.971142\t1.020915\n662\t0.000156\t2.937841\t2.823579\t4.807017\t0.970531\t1.019257\n663\t0.000156\t2.936492\t2.822474\t4.791477\t0.969919\t1.017598\n664\t0.000156\t2.935142\t2.821368\t4.775937\t0.969307\t1.01594\n665\t0.000156\t2.933793\t2.820263\t4.760397\t0.968696\t1.014281\n666\t0.000156\t2.932443\t2.819158\t4.744857\t0.968084\t1.012623\n667\t0.000156\t2.931094\t2.818053\t4.729317\t0.967472\t1.010965\n668\t0.000156\t2.929751\t2.816963\t4.713777\t0.96686\t1.009306\n669\t0.000156\t2.928476\t2.816017\t4.698236\t0.966249\t1.007648\n670\t0.000156\t2.927201\t2.815071\t4.682696\t0.965637\t1.00599\n671\t0.000156\t2.925925\t2.814126\t4.667181\t0.965025\t1.004331\n672\t0.000156\t2.92465\t2.81318\t4.654004\t0.964414\t1.002673\n673\t0.000156\t2.923375\t2.812234\t4.640827\t0.963802\t1.001014\n674\t0.000156\t2.9221\t2.811288\t4.62765\t0.96319\t0.999356\n675\t0.000156\t2.920825\t2.810343\t4.614472\t0.962579\t0.997797\n676\t0.000156\t2.91955\t2.809397\t4.601295\t0.961967\t0.996252\n677\t0.000156\t2.918274\t2.808451\t4.588118\t0.961355\t0.994707\n678\t0.000156\t2.916999\t2.807505\t4.574941\t0.960743\t0.993161\n679\t0.000156\t2.915724\t2.80656\t4.561764\t0.960132\t0.991616\n680\t0.000156\t2.914449\t2.805614\t4.548587\t0.95952\t0.990071\n681\t0.000156\t2.913174\t2.804668\t4.53541\t0.958908\t0.988525\n682\t0.000156\t2.911899\t2.803722\t4.522233\t0.958297\t0.98698\n683\t0.000156\t2.910623\t2.802777\t4.509056\t0.957685\t0.985435\n684\t0.000156\t2.909348\t2.801983\t4.496157\t0.957073\t0.983889\n685\t0.000156\t2.908073\t2.801229\t4.483541\t0.956461\t0.982344\n686\t0.000156\t2.906798\t2.800474\t4.470925\t0.95585\t0.980799\n687\t0.000156\t2.905523\t2.79972\t4.458308\t0.955238\t0.979253\n688\t0.000156\t2.904247\t2.798965\t4.445692\t0.954626\t0.977708\n689\t0.000156\t2.902972\t2.798211\t4.433076\t0.954015\t0.976163\n690\t0.000156\t2.901697\t2.797456\t4.420459\t0.953403\t0.974617\n691\t0.000156\t2.900422\t2.796702\t4.407843\t0.952791\t0.973072\n692\t0.000156\t2.899147\t2.795947\t4.395227\t0.951967\t0.971527\n693\t0.000156\t2.897872\t2.795193\t4.38261\t0.95104\t0.969981\n694\t0.000156\t2.896596\t2.794438\t4.369994\t0.950113\t0.968436\n695\t0.000156\t2.895321\t2.793684\t4.357378\t0.949187\t0.966891\n696\t0.000156\t2.894046\t2.79293\t4.344761\t0.94826\t0.965345\n697\t0.000156\t2.892771\t2.792175\t4.332007\t0.947333\t0.9638\n698\t0.000156\t2.891496\t2.791421\t4.319251\t0.946406\t0.962255\n699\t0.000156\t2.890205\t2.790698\t4.306494\t0.945479\t0.960709\n700\t0.000156\t2.888897\t2.790007\t4.293738\t0.944552\t0.959164\n701\t0.000156\t2.88759\t2.789316\t4.280981\t0.943626\t0.957619\n702\t0.000156\t2.886283\t2.788626\t4.268225\t0.942699\t0.956073\n703\t0.000156\t2.884976\t2.787935\t4.255468\t0.941772\t0.954528\n704\t0.000156\t2.883669\t2.787244\t4.242712\t0.940845\t0.952983\n705\t0.000156\t2.882362\t2.786554\t4.229955\t0.939918\t0.951437\n706\t0.000156\t2.881055\t2.785863\t4.217199\t0.938991\t0.949892\n707\t0.000156\t2.879748\t2.785172\t4.204442\t0.938065\t0.948347\n708\t0.000156\t2.878441\t2.784481\t4.191686\t0.937138\t0.946801\n709\t0.000156\t2.877134\t2.783791\t4.179126\t0.936211\t0.945517\n710\t0.000156\t2.875827\t2.7831\t4.16679\t0.935284\t0.944482\n711\t0.000156\t2.87452\t2.782409\t4.154454\t0.934357\t0.943447\n712\t0.000156\t2.873213\t2.781719\t4.142118\t0.933431\t0.942412\n713\t0.000156\t2.871906\t2.781028\t4.129782\t0.932504\t0.941377\n714\t0.000156\t2.870607\t2.780322\t4.117446\t0.931577\t0.940342\n715\t0.000156\t2.869343\t2.779557\t4.10511\t0.93065\t0.939306\n716\t0.000156\t2.868078\t2.778792\t4.092774\t0.929723\t0.938271\n717\t0.000156\t2.866814\t2.778027\t4.080438\t0.928796\t0.937236\n718\t0.000156\t2.865549\t2.777262\t4.068102\t0.92787\t0.936201\n719\t0.000156\t2.864284\t2.776497\t4.055766\t0.926943\t0.935166\n720\t0.000156\t2.86302\t2.775731\t4.04343\t0.926016\t0.93413\n721\t0.000156\t2.861755\t2.774966\t4.031094\t0.925089\t0.933095\n722\t0.000156\t2.860491\t2.774201\t4.01959\t0.924162\t0.93206\n723\t0.000156\t2.859226\t2.773436\t4.008126\t0.923236\t0.931025\n724\t0.000156\t2.857962\t2.772671\t3.996663\t0.922309\t0.92999\n725\t0.000156\t2.856697\t2.771906\t3.985199\t0.921382\t0.928955\n726\t0.000156\t2.855433\t2.771141\t3.973735\t0.920474\t0.927919\n727\t0.000156\t2.854168\t2.770376\t3.962271\t0.919622\t0.926884\n728\t0.000156\t2.852903\t2.769611\t3.950808\t0.918769\t0.925849\n729\t0.000156\t2.851639\t2.768845\t3.939344\t0.917916\t0.924814\n730\t0.000156\t2.850547\t2.768282\t3.92788\t0.917064\t0.923779\n731\t0.000156\t2.849474\t2.76774\t3.916417\t0.916211\t0.922743\n732\t0.000156\t2.848401\t2.767198\t3.904953\t0.915358\t0.921708\n733\t0.000156\t2.847327\t2.766656\t3.893489\t0.914506\t0.920673\n734\t0.000156\t2.846254\t2.766114\t3.882025\t0.913653\t0.919638\n735\t0.000156\t2.845181\t2.765572\t3.870562\t0.9128\t0.918603\n736\t0.000156\t2.844107\t2.76503\t3.860572\t0.911948\t0.917567\n737\t0.000156\t2.843034\t2.764488\t3.850793\t0.911095\t0.916532\n738\t0.000156\t2.841961\t2.763946\t3.841014\t0.910242\t0.915497\n739\t0.000156\t2.840888\t2.763404\t3.831235\t0.90939\t0.914462\n740\t0.000156\t2.839814\t2.762862\t3.821456\t0.908537\t0.913427\n741\t0.000156\t2.838741\t2.76232\t3.811677\t0.907684\t0.912392\n742\t0.000156\t2.837668\t2.761779\t3.801898\t0.906832\t0.911356\n743\t0.000156\t2.836594\t2.761237\t3.792119\t0.905979\t0.910321\n744\t0.000156\t2.835521\t2.760695\t3.78234\t0.905126\t0.909286\n745\t0.000156\t2.834332\t2.760114\t3.772561\t0.904274\t0.908251\n746\t0.000156\t2.833068\t2.759508\t3.762781\t0.903421\t0.907216\n747\t0.000156\t2.831803\t2.758903\t3.753002\t0.902568\t0.90618\n748\t0.000156\t2.830538\t2.758297\t3.743223\t0.901716\t0.905145\n749\t0.000156\t2.829274\t2.757691\t3.733444\t0.900863\t0.90411\n750\t0.000156\t2.828009\t2.757086\t3.723665\t0.90001\t0.903196\n751\t0.000156\t2.826745\t2.75648\t3.713865\t0.899158\t0.902347\n752\t0.000156\t2.82548\t2.755874\t3.703997\t0.898305\t0.901499\n753\t0.000156\t2.824216\t2.755268\t3.694128\t0.897452\t0.90065\n754\t0.000156\t2.822951\t2.754663\t3.684259\t0.8966\t0.899801\n755\t0.000156\t2.821687\t2.754057\t3.67439\t0.895747\t0.898953\n756\t0.000156\t2.820422\t2.753451\t3.664522\t0.894894\t0.898104\n757\t0.000156\t2.819157\t2.752846\t3.654653\t0.894042\t0.897255\n758\t0.000156\t2.817893\t2.75224\t3.644784\t0.893189\t0.896407\n759\t0.000156\t2.816628\t2.751634\t3.634915\t0.892336\t0.895558\n760\t0.000156\t2.815357\t2.750979\t3.625046\t0.891484\t0.89471\n761\t0.000156\t2.814071\t2.750214\t3.615178\t0.890694\t0.893861\n762\t0.000156\t2.812786\t2.749449\t3.605309\t0.889915\t0.893012\n763\t0.000156\t2.8115\t2.748684\t3.59544\t0.889137\t0.892164\n764\t0.000156\t2.810214\t2.747919\t3.585571\t0.888358\t0.891315\n765\t0.000156\t2.808928\t2.747154\t3.575703\t0.88758\t0.890466\n766\t0.000156\t2.807642\t2.746389\t3.565834\t0.886801\t0.889618\n767\t0.000156\t2.806357\t2.745624\t3.555965\t0.886022\t0.888769\n768\t0.000156\t2.805071\t2.744859\t3.546096\t0.885244\t0.88792\n769\t0.000156\t2.803785\t2.744093\t3.536228\t0.884465\t0.887072\n770\t0.000156\t2.802499\t2.743328\t3.526359\t0.883687\t0.886223\n771\t0.000156\t2.801213\t2.742563\t3.51649\t0.882908\t0.885374\n772\t0.000156\t2.799928\t2.741798\t3.506621\t0.88213\t0.884526\n773\t0.000156\t2.798642\t2.741033\t3.496752\t0.881351\t0.883677\n774\t0.000156\t2.797356\t2.740268\t3.486884\t0.880573\t0.882828\n775\t0.000156\t2.796072\t2.739505\t3.477015\t0.879794\t0.88198\n776\t0.000156\t2.794988\t2.738974\t3.467146\t0.879016\t0.881131\n777\t0.000156\t2.793904\t2.738442\t3.457277\t0.878237\t0.880282\n778\t0.000156\t2.79282\t2.737911\t3.447409\t0.877459\t0.879434\n779\t0.000156\t2.791736\t2.73738\t3.43754\t0.87668\t0.878585\n780\t0.000156\t2.790653\t2.736848\t3.427671\t0.875902\t0.877736\n781\t0.000156\t2.789569\t2.736317\t3.417802\t0.875123\t0.876888\n782\t0.000156\t2.788485\t2.735786\t3.407934\t0.874345\t0.876039\n783\t0.000156\t2.787401\t2.735254\t3.39903\t0.873566\t0.87519\n784\t0.000156\t2.786317\t2.734723\t3.390181\t0.872787\t0.874342\n785\t0.000156\t2.785233\t2.734192\t3.381331\t0.872009\t0.873493\n786\t0.000156\t2.784149\t2.73366\t3.372482\t0.87123\t0.872644\n787\t0.000156\t2.783065\t2.733129\t3.363633\t0.870452\t0.871796\n788\t0.000156\t2.781981\t2.732598\t3.354784\t0.869673\t0.870947\n789\t0.000156\t2.780897\t2.732066\t3.345934\t0.868895\t0.870098\n790\t0.000156\t2.779814\t2.731535\t3.337085\t0.868116\t0.86925\n791\t0.000156\t2.778828\t2.73111\t3.328236\t0.867338\t0.868401\n792\t0.000156\t2.777882\t2.730727\t3.319386\t0.866559\t0.867552\n793\t0.000156\t2.776936\t2.730345\t3.310537\t0.865781\t0.866704\n794\t0.000156\t2.775991\t2.729962\t3.301688\t0.865002\t0.865855\n795\t0.000156\t2.775045\t2.729579\t3.292839\t0.864272\t0.865006\n796\t0.000156\t2.774099\t2.729197\t3.283989\t0.863604\t0.864158\n797\t0.000156\t2.773153\t2.728814\t3.27514\t0.862937\t0.863309\n798\t0.000156\t2.772208\t2.728432\t3.266291\t0.86227\t0.86246\n799\t0.000156\t2.771262\t2.728049\t3.257442\t0.861603\t0.861612\n800\t0.000156\t2.770316\t2.727667\t3.249322\t0.860935\t0.860763\n801\t0.000156\t2.76937\t2.727284\t3.24146\t0.860268\t0.859914\n802\t0.000156\t2.768425\t2.726902\t3.233597\t0.859601\t0.859066\n803\t0.000156\t2.767479\t2.726519\t3.225735\t0.858933\t0.858217\n804\t0.000156\t2.766533\t2.726136\t3.217872\t0.858266\t0.857368\n805\t0.000156\t2.765587\t2.725754\t3.21001\t0.857599\t0.85652\n806\t0.000156\t2.764628\t2.725323\t3.202147\t0.856931\t0.855671\n807\t0.000156\t2.763651\t2.724824\t3.194285\t0.856264\t0.854822\n808\t0.000156\t2.762673\t2.724324\t3.186422\t0.855597\t0.853974\n809\t0.000156\t2.761695\t2.723825\t3.17856\t0.854929\t0.853125\n810\t0.000156\t2.760718\t2.723325\t3.170697\t0.854262\t0.852276\n811\t0.000156\t2.75974\t2.722826\t3.162835\t0.853595\t0.851428\n812\t0.000156\t2.758763\t2.722326\t3.154972\t0.852928\t0.850579\n813\t0.000156\t2.757785\t2.721827\t3.14711\t0.85226\t0.84973\n814\t0.000156\t2.756807\t2.721327\t3.139247\t0.851593\t0.848882\n815\t0.000156\t2.75583\t2.720828\t3.131385\t0.850926\t0.848033\n816\t0.000156\t2.754852\t2.720329\t3.123523\t0.850258\t0.847184\n817\t0.000156\t2.753874\t2.719829\t3.11566\t0.849591\t0.846336\n818\t0.000156\t2.752897\t2.71933\t3.107798\t0.848924\t0.845487\n819\t0.000156\t2.751919\t2.71883\t3.099935\t0.848256\t0.844638\n820\t0.000156\t2.750941\t2.718331\t3.092176\t0.847589\t0.84379\n821\t0.000156\t2.749956\t2.717831\t3.084568\t0.846922\t0.842941\n822\t0.000156\t2.748915\t2.717332\t3.07696\t0.846254\t0.842092\n823\t0.000156\t2.747874\t2.716832\t3.069352\t0.845587\t0.841244\n824\t0.000156\t2.746832\t2.716333\t3.061744\t0.84492\t0.840395\n825\t0.000156\t2.745791\t2.715834\t3.054137\t0.844252\t0.839546\n826\t0.000156\t2.744749\t2.715334\t3.046529\t0.843585\t0.838698\n827\t0.000156\t2.743708\t2.714835\t3.038921\t0.842918\t0.837876\n828\t0.000156\t2.742667\t2.714335\t3.031313\t0.842251\t0.837257\n829\t0.000156\t2.741625\t2.713836\t3.023705\t0.841585\t0.836638\n830\t0.000156\t2.740584\t2.713336\t3.016098\t0.840991\t0.83602\n831\t0.000156\t2.739542\t2.712837\t3.00849\t0.840398\t0.835401\n832\t0.000156\t2.738501\t2.712337\t3.000882\t0.839805\t0.834782\n833\t0.000156\t2.73746\t2.711838\t2.993274\t0.839212\t0.834163\n834\t0.000156\t2.736418\t2.711339\t2.985666\t0.838619\t0.833545\n835\t0.000156\t2.735377\t2.710839\t2.978059\t0.838026\t0.832926\n836\t0.000156\t2.734335\t2.71034\t2.970451\t0.837432\t0.832307\n837\t0.000156\t2.733381\t2.709675\t2.962843\t0.836839\t0.831688\n838\t0.000156\t2.732446\t2.708974\t2.955235\t0.836246\t0.83107\n839\t0.000156\t2.731511\t2.708272\t2.947627\t0.835653\t0.830451\n840\t0.000156\t2.730576\t2.707571\t2.940057\t0.83506\t0.829832\n841\t0.000156\t2.72964\t2.70687\t2.932995\t0.834467\t0.829214\n842\t0.000156\t2.728705\t2.706168\t2.925932\t0.833873\t0.828595\n843\t0.000156\t2.72777\t2.705467\t2.91887\t0.83328\t0.827976\n844\t0.000156\t2.726835\t2.704766\t2.911807\t0.832687\t0.827357\n845\t0.000156\t2.7259\t2.704064\t2.904745\t0.832094\t0.826739\n846\t0.000156\t2.724965\t2.703363\t2.897682\t0.831501\t0.82612\n847\t0.000156\t2.72403\t2.702662\t2.89062\t0.830908\t0.825501\n848\t0.000156\t2.723094\t2.70196\t2.883557\t0.830314\t0.824882\n849\t0.000156\t2.722159\t2.701259\t2.876495\t0.829721\t0.824264\n850\t0.000156\t2.721224\t2.700558\t2.869432\t0.829128\t0.823645\n851\t0.000156\t2.720289\t2.699856\t2.86237\t0.828535\t0.823026\n852\t0.000156\t2.719277\t2.69932\t2.855307\t0.827942\t0.822408\n853\t0.000156\t2.718193\t2.698936\t2.848245\t0.827349\t0.821789\n854\t0.000156\t2.717109\t2.698552\t2.841182\t0.826756\t0.82117\n855\t0.000156\t2.716025\t2.698167\t2.83412\t0.826162\t0.820551\n856\t0.000156\t2.714941\t2.697783\t2.827057\t0.825569\t0.819933\n857\t0.000156\t2.713857\t2.697399\t2.819995\t0.824976\t0.819314\n858\t0.000156\t2.712773\t2.697015\t2.812932\t0.824383\t0.818695\n859\t0.000156\t2.711689\t2.696631\t2.80587\t0.82379\t0.818076\n860\t0.000156\t2.710605\t2.696247\t2.798808\t0.823197\t0.817458\n861\t0.000156\t2.709521\t2.695863\t2.791745\t0.822603\t0.816839\n862\t0.000156\t2.708438\t2.695525\t2.784851\t0.82201\t0.81622\n863\t0.000156\t2.707354\t2.695201\t2.778788\t0.821417\t0.815601\n864\t0.000156\t2.70627\t2.694876\t2.772725\t0.820757\t0.814983\n865\t0.000156\t2.705186\t2.694551\t2.766663\t0.820052\t0.814364\n866\t0.000156\t2.704102\t2.694226\t2.7606\t0.819348\t0.813745\n867\t0.000156\t2.703053\t2.693902\t2.754537\t0.818644\t0.813127\n868\t0.000156\t2.702129\t2.693577\t2.748474\t0.817939\t0.812508\n869\t0.000156\t2.701204\t2.693252\t2.742411\t0.817235\t0.811889\n870\t0.000156\t2.70028\t2.692927\t2.736348\t0.81653\t0.81127\n871\t0.000156\t2.699355\t2.692603\t2.730286\t0.815826\t0.810652\n872\t0.000156\t2.698431\t2.692278\t2.724223\t0.815122\t0.810033\n873\t0.000156\t2.697506\t2.691953\t2.71816\t0.814417\t0.809414\n874\t0.000207\t2.696582\t2.691628\t2.712097\t0.813713\t0.808795\n875\t0.000395\t2.695657\t2.691243\t2.706034\t0.813008\t0.808177\n876\t0.000584\t2.694733\t2.690729\t2.699971\t0.812304\t0.807558\n877\t0.000773\t2.693808\t2.690215\t2.693908\t0.8116\t0.806939\n878\t0.000962\t2.692884\t2.689701\t2.687846\t0.810895\t0.80632\n879\t0.00115\t2.691959\t2.689186\t2.681783\t0.810191\t0.805702\n880\t0.001339\t2.691035\t2.688672\t2.67572\t0.809487\t0.805083\n881\t0.001528\t2.69011\t2.688158\t2.669657\t0.808782\t0.804464\n882\t0.001717\t2.689186\t2.687643\t2.663594\t0.808078\t0.803846\n883\t0.001905\t2.688104\t2.687129\t2.657531\t0.807373\t0.803227\n884\t0.002094\t2.68701\t2.686615\t2.651469\t0.806669\t0.802608\n885\t0.002283\t2.685915\t2.6861\t2.645406\t0.805965\t0.801989\n886\t0.002472\t2.684821\t2.685586\t2.639343\t0.80526\t0.801371\n887\t0.00266\t2.683726\t2.685072\t2.633304\t0.804556\t0.800752\n888\t0.002849\t2.682632\t2.68452\t2.627411\t0.803851\t0.800192\n889\t0.003038\t2.681537\t2.683948\t2.621518\t0.803147\t0.799744\n890\t0.003123\t2.680443\t2.683377\t2.615624\t0.802443\t0.799295\n891\t0.003204\t2.679348\t2.682805\t2.609731\t0.801738\t0.798847\n892\t0.003286\t2.678253\t2.682234\t2.603838\t0.801034\t0.798398\n893\t0.003367\t2.677159\t2.681662\t2.597945\t0.80033\t0.797949\n894\t0.003449\t2.676064\t2.681091\t2.592052\t0.799625\t0.797501\n895\t0.003531\t2.67497\t2.680519\t2.586159\t0.798921\t0.797052\n896\t0.003612\t2.673875\t2.679948\t2.580266\t0.798216\t0.796604\n897\t0.003694\t2.672781\t2.679376\t2.574373\t0.797512\t0.796155\n898\t0.003776\t2.671626\t2.678805\t2.56848\t0.796836\t0.795707\n899\t0.003857\t2.670436\t2.67833\t2.562586\t0.79628\t0.795258\n900\t0.003939\t2.669246\t2.67812\t2.556693\t0.795724\t0.794809\n901\t0.00402\t2.668056\t2.67791\t2.5508\t0.795168\t0.794361\n902\t0.004102\t2.666866\t2.6777\t2.544907\t0.794611\t0.793912\n903\t0.004184\t2.665676\t2.67749\t2.539014\t0.794055\t0.793464\n904\t0.004265\t2.664485\t2.67728\t2.533121\t0.793499\t0.793015\n905\t0.004299\t2.663295\t2.67707\t2.527228\t0.792943\t0.792566\n906\t0.004309\t2.662105\t2.67686\t2.521335\t0.792387\t0.792118\n907\t0.004319\t2.660915\t2.67665\t2.515441\t0.791831\t0.791669\n908\t0.004329\t2.659725\t2.67644\t2.509548\t0.791275\t0.791221\n909\t0.00434\t2.658535\t2.676231\t2.503655\t0.790719\t0.790772\n910\t0.00435\t2.657344\t2.676021\t2.497762\t0.790163\t0.790324\n911\t0.00436\t2.656154\t2.675811\t2.491869\t0.789607\t0.789875\n912\t0.00437\t2.654964\t2.675601\t2.485976\t0.789051\t0.789426\n913\t0.004381\t2.653788\t2.675258\t2.480083\t0.788494\t0.788978\n914\t0.004391\t2.65264\t2.674642\t2.474422\t0.787938\t0.788529\n915\t0.004401\t2.651493\t2.674025\t2.468952\t0.787382\t0.788081\n916\t0.004411\t2.650345\t2.673409\t2.463482\t0.786826\t0.787632\n917\t0.004421\t2.649197\t2.672792\t2.458013\t0.78627\t0.787184\n918\t0.004432\t2.64805\t2.672176\t2.452543\t0.785714\t0.786735\n919\t0.004442\t2.646902\t2.67156\t2.447074\t0.785158\t0.786286\n920\t0.004498\t2.645754\t2.670943\t2.441604\t0.784602\t0.785838\n921\t0.00463\t2.644607\t2.670327\t2.436135\t0.784046\t0.785389\n922\t0.004763\t2.643459\t2.669711\t2.430665\t0.78349\t0.784941\n923\t0.004896\t2.642311\t2.669094\t2.425196\t0.782934\t0.784492\n924\t0.005028\t2.641164\t2.668478\t2.419726\t0.782377\t0.784043\n925\t0.005161\t2.640016\t2.667862\t2.414257\t0.781821\t0.783595\n926\t0.005293\t2.638868\t2.667245\t2.408787\t0.781265\t0.783146\n927\t0.005426\t2.637721\t2.666629\t2.403318\t0.780709\t0.782698\n928\t0.005559\t2.636573\t2.666024\t2.397848\t0.780153\t0.782249\n929\t0.005691\t2.635436\t2.665801\t2.392379\t0.779597\t0.781801\n930\t0.005824\t2.634299\t2.665578\t2.386909\t0.779041\t0.781352\n931\t0.005957\t2.633162\t2.665355\t2.381439\t0.778485\t0.780903\n932\t0.006089\t2.632025\t2.665132\t2.37597\t0.777929\t0.780455\n933\t0.006222\t2.630888\t2.664909\t2.3705\t0.777401\t0.780006\n934\t0.006355\t2.629751\t2.664685\t2.365031\t0.776882\t0.779558\n935\t0.006507\t2.628614\t2.664462\t2.359561\t0.776363\t0.779109\n936\t0.006894\t2.627477\t2.664239\t2.354092\t0.775844\t0.77866\n937\t0.007282\t2.62634\t2.664016\t2.348622\t0.775325\t0.778212\n938\t0.00767\t2.625203\t2.663793\t2.343153\t0.774806\t0.777763\n939\t0.008057\t2.624066\t2.66357\t2.337683\t0.774287\t0.777315\n940\t0.008445\t2.622929\t2.663347\t2.332214\t0.773768\t0.776866\n941\t0.008833\t2.621792\t2.663123\t2.326744\t0.773249\t0.776418\n942\t0.00922\t2.620655\t2.6629\t2.321275\t0.77273\t0.775969\n943\t0.009608\t2.619518\t2.662677\t2.315805\t0.772211\t0.77552\n944\t0.009996\t2.618334\t2.662407\t2.310741\t0.771692\t0.775072\n945\t0.010383\t2.617133\t2.66212\t2.305761\t0.771173\t0.774623\n946\t0.010771\t2.615932\t2.661833\t2.300782\t0.770654\t0.774175\n947\t0.011159\t2.614732\t2.661547\t2.295803\t0.770135\t0.773726\n948\t0.011546\t2.613531\t2.66126\t2.290824\t0.769616\t0.773278\n949\t0.011934\t2.61233\t2.660973\t2.285844\t0.769097\t0.772829\n950\t0.012322\t2.611129\t2.660686\t2.280865\t0.768578\t0.77238\n951\t0.01265\t2.609928\t2.660399\t2.275886\t0.768059\t0.771962\n952\t0.012961\t2.608728\t2.660112\t2.270907\t0.76754\t0.771575\n953\t0.013272\t2.607527\t2.659825\t2.265927\t0.767021\t0.771188\n954\t0.013583\t2.606326\t2.659538\t2.260948\t0.766502\t0.770802\n955\t0.013895\t2.605125\t2.659251\t2.255969\t0.765983\t0.770415\n956\t0.014206\t2.603924\t2.658964\t2.25099\t0.765464\t0.770028\n957\t0.014517\t2.602724\t2.658677\t2.24601\t0.764945\t0.769641\n958\t0.014828\t2.601523\t2.65839\t2.241031\t0.764426\t0.769255\n959\t0.015139\t2.6004\t2.658163\t2.236052\t0.763907\t0.768868\n960\t0.01545\t2.59938\t2.658015\t2.231073\t0.763388\t0.768481\n961\t0.015762\t2.59836\t2.657866\t2.226094\t0.762869\t0.768095\n962\t0.016073\t2.59734\t2.657717\t2.221114\t0.76235\t0.767708\n963\t0.016384\t2.59632\t2.657568\t2.216135\t0.761831\t0.767321\n964\t0.016695\t2.5953\t2.65742\t2.211156\t0.761312\t0.766934\n965\t0.017006\t2.59428\t2.657271\t2.206177\t0.760793\t0.766548\n966\t0.017173\t2.593259\t2.657122\t2.201197\t0.760274\t0.766161\n967\t0.017183\t2.592239\t2.656973\t2.196218\t0.759795\t0.765774\n968\t0.017193\t2.591219\t2.656825\t2.191239\t0.759387\t0.765388\n969\t0.017204\t2.590199\t2.656676\t2.18626\t0.758979\t0.765001\n970\t0.017214\t2.589179\t2.656527\t2.18128\t0.758572\t0.764614\n971\t0.017224\t2.588159\t2.656378\t2.176301\t0.758164\t0.764228\n972\t0.017234\t2.587139\t2.656229\t2.171322\t0.757756\t0.763841\n973\t0.017244\t2.586118\t2.656081\t2.166343\t0.757348\t0.763454\n974\t0.017255\t2.585094\t2.655886\t2.161363\t0.75694\t0.763067\n975\t0.017265\t2.584042\t2.655397\t2.156753\t0.756533\t0.762681\n976\t0.017275\t2.58299\t2.654908\t2.152455\t0.756125\t0.762294\n977\t0.017285\t2.581938\t2.654419\t2.148158\t0.755717\t0.761907\n978\t0.017295\t2.580886\t2.65393\t2.14386\t0.755309\t0.761521\n979\t0.017306\t2.579834\t2.653442\t2.139563\t0.754901\t0.761134\n980\t0.017316\t2.578782\t2.652953\t2.135266\t0.754494\t0.760747\n981\t0.017305\t2.57773\t2.652464\t2.130968\t0.754086\t0.76036\n982\t0.017198\t2.576678\t2.651975\t2.126671\t0.753678\t0.759974\n983\t0.01709\t2.575626\t2.651486\t2.122373\t0.75327\t0.759587\n984\t0.016983\t2.574574\t2.650998\t2.118076\t0.752862\t0.7592\n985\t0.016876\t2.573522\t2.650509\t2.113778\t0.752455\t0.758814\n986\t0.016769\t2.57247\t2.65002\t2.109481\t0.752047\t0.758427\n987\t0.016662\t2.571418\t2.649531\t2.105183\t0.751639\t0.75804\n988\t0.016555\t2.570366\t2.649042\t2.100886\t0.751231\t0.757654\n989\t0.016448\t2.569314\t2.648553\t2.096589\t0.750823\t0.757267\n990\t0.016341\t2.568279\t2.648127\t2.092291\t0.750416\t0.75688\n991\t0.016233\t2.567249\t2.647713\t2.087994\t0.750008\t0.756493\n992\t0.016126\t2.566218\t2.647298\t2.083696\t0.7496\t0.756107\n993\t0.016019\t2.565187\t2.646884\t2.079399\t0.749192\t0.75572\n994\t0.015912\t2.564156\t2.646469\t2.075101\t0.748784\t0.755333\n995\t0.015805\t2.563126\t2.646055\t2.070804\t0.748377\t0.754947\n996\t0.015698\t2.562095\t2.64564\t2.066507\t0.747969\t0.75456\n997\t0.015514\t2.561064\t2.645226\t2.062209\t0.747561\t0.754173\n998\t0.01532\t2.560033\t2.644811\t2.057912\t0.747153\t0.753786\n999\t0.015126\t2.559002\t2.644397\t2.053614\t0.746745\t0.7534\n1000\t0.014933\t2.557972\t2.643983\t2.049317\t0.746338\t0.753013\n1001\t0.014739\t2.556941\t2.643568\t2.045019\t0.74593\t0.752626\n1002\t0.014545\t2.55591\t2.643154\t2.040722\t0.745487\t0.75224\n1003\t0.014351\t2.554879\t2.642739\t2.036424\t0.745042\t0.751853\n1004\t0.014157\t2.553849\t2.642325\t2.032127\t0.744597\t0.751466\n1005\t0.013963\t2.552783\t2.641882\t2.02783\t0.744152\t0.751079\n1006\t0.013769\t2.551689\t2.641414\t2.023532\t0.743707\t0.750693\n1007\t0.013576\t2.550594\t2.640947\t2.019235\t0.743263\t0.750306\n1008\t0.013382\t2.5495\t2.640479\t2.015166\t0.742818\t0.749919\n1009\t0.013188\t2.548405\t2.640011\t2.011199\t0.742373\t0.749533\n1010\t0.012994\t2.547311\t2.639544\t2.007232\t0.741928\t0.749146\n1011\t0.0128\t2.546216\t2.639076\t2.003265\t0.741483\t0.748759\n1012\t0.0126\t2.545122\t2.638609\t1.999299\t0.741038\t0.748621\n1013\t0.012396\t2.544027\t2.638141\t1.995332\t0.740593\t0.748584\n1014\t0.012192\t2.542933\t2.637674\t1.991365\t0.740148\t0.748546\n1015\t0.011988\t2.541838\t2.637206\t1.987398\t0.739704\t0.748508\n1016\t0.011784\t2.540744\t2.636739\t1.983431\t0.739259\t0.74847\n1017\t0.01158\t2.539649\t2.636271\t1.979465\t0.738814\t0.748432\n1018\t0.011376\t2.538554\t2.635803\t1.975498\t0.738369\t0.748394\n1019\t0.011172\t2.53746\t2.635336\t1.971531\t0.737924\t0.748356\n1020\t0.010968\t2.536383\t2.634861\t1.967564\t0.737479\t0.748318\n1021\t0.010764\t2.535363\t2.634361\t1.963597\t0.737034\t0.74828\n1022\t0.01056\t2.534343\t2.633862\t1.959631\t0.736589\t0.748243\n1023\t0.010356\t2.533323\t2.633362\t1.955664\t0.736145\t0.748205\n1024\t0.010152\t2.532303\t2.632863\t1.951697\t0.7357\t0.748167\n1025\t0.009948\t2.531283\t2.632363\t1.94773\t0.735255\t0.748129\n1026\t0.009744\t2.530263\t2.631864\t1.943764\t0.73481\t0.748091\n1027\t0.009546\t2.529242\t2.631364\t1.939797\t0.734365\t0.748053\n1028\t0.009362\t2.528222\t2.630865\t1.93583\t0.73392\t0.748015\n1029\t0.009178\t2.527202\t2.630366\t1.931863\t0.733475\t0.747977\n1030\t0.008995\t2.526182\t2.629866\t1.927896\t0.73303\t0.747939\n1031\t0.008811\t2.525162\t2.629367\t1.92393\t0.732586\t0.747901\n1032\t0.008627\t2.524142\t2.628867\t1.919963\t0.732141\t0.747864\n1033\t0.008444\t2.523122\t2.628368\t1.915996\t0.731696\t0.747826\n1034\t0.00826\t2.522101\t2.627868\t1.912029\t0.731251\t0.747788\n1035\t0.008077\t2.521081\t2.627369\t1.908062\t0.730806\t0.74775\n1036\t0.007893\t2.520051\t2.62691\t1.904096\t0.730351\t0.747712\n1037\t0.007709\t2.51902\t2.626453\t1.900129\t0.729888\t0.747674\n1038\t0.007526\t2.51799\t2.625996\t1.896162\t0.729424\t0.747636\n1039\t0.007342\t2.516959\t2.625539\t1.892195\t0.728961\t0.747598\n1040\t0.007158\t2.515928\t2.625082\t1.888229\t0.728498\t0.74756\n1041\t0.006975\t2.514897\t2.624625\t1.884262\t0.728034\t0.747522\n1042\t0.006791\t2.513866\t2.624168\t1.880459\t0.727571\t0.747485\n1043\t0.006643\t2.512836\t2.623711\t1.877086\t0.727107\t0.747447\n1044\t0.006495\t2.511805\t2.623254\t1.873712\t0.726644\t0.747409\n1045\t0.006347\t2.510774\t2.622797\t1.870338\t0.726181\t0.747371\n1046\t0.006199\t2.509743\t2.62234\t1.866965\t0.725717\t0.747333\n1047\t0.006051\t2.508713\t2.621883\t1.863591\t0.725254\t0.747295\n1048\t0.005903\t2.507682\t2.621426\t1.860217\t0.72479\t0.747257\n1049\t0.005755\t2.506651\t2.620969\t1.856844\t0.724327\t0.747219\n1050\t0.005607\t2.50562\t2.620512\t1.85347\t0.723864\t0.747181\n1051\t0.005459\t2.504603\t2.620062\t1.850097\t0.7234\t0.747144\n1052\t0.005311\t2.503594\t2.619616\t1.846723\t0.722937\t0.747106\n1053\t0.005163\t2.502584\t2.61917\t1.843349\t0.722473\t0.747068\n1054\t0.005015\t2.501575\t2.618723\t1.839976\t0.72201\t0.74703\n1055\t0.004868\t2.500565\t2.618277\t1.836602\t0.721547\t0.746992\n1056\t0.00472\t2.499556\t2.617831\t1.833228\t0.721083\t0.746954\n1057\t0.004572\t2.498546\t2.617384\t1.829855\t0.72062\t0.746916\n1058\t0.004508\t2.497537\t2.616938\t1.826481\t0.720156\t0.746878\n1059\t0.004483\t2.496527\t2.616492\t1.823108\t0.719693\t0.74684\n1060\t0.004457\t2.495518\t2.616045\t1.819734\t0.719229\t0.746802\n1061\t0.004432\t2.494508\t2.615599\t1.81636\t0.718766\t0.746765\n1062\t0.004406\t2.493499\t2.615153\t1.812987\t0.718303\t0.746727\n1063\t0.004381\t2.492489\t2.614707\t1.809613\t0.717839\t0.746689\n1064\t0.004355\t2.491479\t2.61426\t1.806239\t0.717376\t0.746651\n1065\t0.00433\t2.49047\t2.613814\t1.802866\t0.716912\t0.746613\n1066\t0.004304\t2.489505\t2.61343\t1.799492\t0.716449\t0.746575\n1067\t0.004279\t2.488623\t2.613165\t1.796119\t0.715986\t0.746451\n1068\t0.004253\t2.487741\t2.612899\t1.792745\t0.715522\t0.746064\n1069\t0.004228\t2.486859\t2.612633\t1.789371\t0.715059\t0.745678\n1070\t0.004202\t2.485977\t2.612368\t1.785998\t0.714591\t0.745292\n1071\t0.004177\t2.485095\t2.612102\t1.782624\t0.71409\t0.744905\n1072\t0.004151\t2.484213\t2.611836\t1.779251\t0.71359\t0.744519\n1073\t0.00416\t2.483331\t2.611571\t1.775877\t0.713089\t0.744133\n1074\t0.004221\t2.482449\t2.611305\t1.772503\t0.712589\t0.743746\n1075\t0.004283\t2.481567\t2.611039\t1.76913\t0.712089\t0.74336\n1076\t0.004344\t2.480685\t2.610774\t1.765756\t0.711588\t0.742974\n1077\t0.004405\t2.479803\t2.610508\t1.762462\t0.711088\t0.742587\n1078\t0.004466\t2.478921\t2.610242\t1.759181\t0.710587\t0.742201\n1079\t0.004527\t2.478039\t2.609977\t1.7559\t0.710087\t0.741815\n1080\t0.004589\t2.477157\t2.609711\t1.75262\t0.709586\t0.741428\n1081\t0.00465\t2.476273\t2.609439\t1.749339\t0.709086\t0.741042\n1082\t0.004711\t2.475348\t2.609035\t1.746058\t0.708585\t0.740656\n1083\t0.004772\t2.474424\t2.608631\t1.742777\t0.708085\t0.740269\n1084\t0.004833\t2.473499\t2.608227\t1.739496\t0.707584\t0.739883\n1085\t0.004895\t2.472575\t2.607823\t1.736215\t0.707084\t0.739497\n1086\t0.004956\t2.47165\t2.60742\t1.732934\t0.706583\t0.73911\n1087\t0.005017\t2.470726\t2.607016\t1.729653\t0.706083\t0.738724\n1088\t0.005085\t2.469801\t2.606612\t1.726372\t0.705582\t0.738338\n1089\t0.005212\t2.468877\t2.606208\t1.723091\t0.705082\t0.737951\n1090\t0.00534\t2.467952\t2.605804\t1.71981\t0.704581\t0.737565\n1091\t0.005467\t2.467028\t2.605401\t1.716529\t0.704081\t0.737178\n1092\t0.005595\t2.466103\t2.604997\t1.713248\t0.70358\t0.736792\n1093\t0.005722\t2.465179\t2.604593\t1.709967\t0.70308\t0.736406\n1094\t0.00585\t2.464254\t2.604189\t1.706686\t0.702579\t0.736019\n1095\t0.005977\t2.46333\t2.603785\t1.703405\t0.702079\t0.735633\n1096\t0.006105\t2.462405\t2.603382\t1.700125\t0.701578\t0.735247\n1097\t0.006232\t2.461481\t2.603082\t1.696844\t0.701078\t0.73486\n1098\t0.00636\t2.460556\t2.602816\t1.693563\t0.700577\t0.734474\n1099\t0.006487\t2.459632\t2.60255\t1.690282\t0.700077\t0.734088\n1100\t0.006615\t2.458707\t2.602285\t1.687001\t0.699576\t0.733701\n1101\t0.006743\t2.457783\t2.602019\t1.68372\t0.699076\t0.733315\n1102\t0.00687\t2.456858\t2.601753\t1.680439\t0.698576\t0.732929\n1103\t0.006998\t2.455934\t2.601488\t1.677158\t0.698075\t0.732542\n1104\t0.007097\t2.455009\t2.601222\t1.673877\t0.697575\t0.732156\n1105\t0.007188\t2.454085\t2.600956\t1.670596\t0.697231\t0.73177\n1106\t0.00728\t2.45316\t2.600691\t1.667315\t0.696953\t0.731383\n1107\t0.007372\t2.452236\t2.600425\t1.664034\t0.696675\t0.730997\n1108\t0.007464\t2.451311\t2.600159\t1.660753\t0.696397\t0.730611\n1109\t0.007556\t2.450387\t2.599894\t1.657472\t0.696119\t0.730224\n1110\t0.007648\t2.449462\t2.599628\t1.654191\t0.695841\t0.729838\n1111\t0.007739\t2.448537\t2.599362\t1.651085\t0.695563\t0.729452\n1112\t0.007831\t2.447652\t2.599217\t1.648193\t0.695285\t0.729065\n1113\t0.007923\t2.446812\t2.599217\t1.645302\t0.695007\t0.728679\n1114\t0.008015\t2.445973\t2.599217\t1.64241\t0.694729\t0.728293\n1115\t0.008107\t2.445133\t2.599217\t1.639518\t0.694451\t0.727906\n1116\t0.008198\t2.444294\t2.599217\t1.636627\t0.694173\t0.72752\n1117\t0.00829\t2.443454\t2.599217\t1.633735\t0.693895\t0.727134\n1118\t0.008382\t2.442615\t2.599217\t1.630843\t0.693616\t0.726747\n1119\t0.008683\t2.441775\t2.599217\t1.627952\t0.693338\t0.726361\n1120\t0.009193\t2.440936\t2.599217\t1.62506\t0.69306\t0.725975\n1121\t0.009703\t2.440096\t2.599217\t1.622168\t0.692782\t0.725588\n1122\t0.010213\t2.439257\t2.599217\t1.619277\t0.692504\t0.725202\n1123\t0.010724\t2.438417\t2.599217\t1.616385\t0.692226\t0.724816\n1124\t0.011234\t2.437578\t2.599217\t1.613493\t0.691948\t0.724429\n1125\t0.011744\t2.436738\t2.599217\t1.610602\t0.69167\t0.724043\n1126\t0.012254\t2.435899\t2.599217\t1.60771\t0.691392\t0.723657\n1127\t0.012764\t2.435061\t2.59929\t1.604818\t0.691114\t0.72327\n1128\t0.013274\t2.434232\t2.599758\t1.601927\t0.690836\t0.722884\n1129\t0.013784\t2.433403\t2.600225\t1.599035\t0.690558\t0.722498\n1130\t0.014294\t2.432574\t2.600693\t1.596143\t0.69028\t0.722111\n1131\t0.014805\t2.431745\t2.60116\t1.593252\t0.690002\t0.721725\n1132\t0.015315\t2.430916\t2.601628\t1.59036\t0.689724\t0.721339\n1133\t0.015825\t2.430088\t2.602095\t1.587468\t0.689446\t0.720952\n1134\t0.016442\t2.429259\t2.602563\t1.584577\t0.689168\t0.720566\n1135\t0.017483\t2.42843\t2.603031\t1.581685\t0.68889\t0.72018\n1136\t0.018523\t2.427601\t2.603498\t1.578793\t0.688612\t0.719793\n1137\t0.019564\t2.426772\t2.603966\t1.575901\t0.688334\t0.719407\n1138\t0.020605\t2.425943\t2.604433\t1.57301\t0.688056\t0.719021\n1139\t0.021645\t2.425114\t2.604901\t1.570118\t0.687702\t0.718634\n1140\t0.022686\t2.424286\t2.605368\t1.567226\t0.687164\t0.718248\n1141\t0.023727\t2.423457\t2.605836\t1.564335\t0.686627\t0.717862\n1142\t0.024767\t2.422628\t2.606304\t1.561443\t0.686089\t0.717475\n1143\t0.025808\t2.421826\t2.606899\t1.558551\t0.685552\t0.717089\n1144\t0.026848\t2.421029\t2.607515\t1.55566\t0.685014\t0.716703\n1145\t0.027889\t2.420232\t2.608131\t1.552772\t0.684476\t0.716316\n1146\t0.02893\t2.419435\t2.608748\t1.549991\t0.683939\t0.71593\n1147\t0.02997\t2.418638\t2.609364\t1.547211\t0.683401\t0.715544\n1148\t0.031011\t2.417841\t2.60998\t1.544431\t0.682864\t0.715157\n1149\t0.032052\t2.417044\t2.610597\t1.54165\t0.682326\t0.714771\n1150\t0.032622\t2.416247\t2.611213\t1.53887\t0.681789\t0.714385\n1151\t0.033142\t2.41545\t2.611829\t1.536089\t0.681251\t0.713998\n1152\t0.033662\t2.414653\t2.612446\t1.533309\t0.680714\t0.713612\n1153\t0.034183\t2.413856\t2.613062\t1.530528\t0.680176\t0.713226\n1154\t0.034703\t2.413059\t2.613678\t1.527748\t0.679638\t0.712839\n1155\t0.035223\t2.412262\t2.614295\t1.524967\t0.679101\t0.712453\n1156\t0.035744\t2.411465\t2.614911\t1.522187\t0.678563\t0.712067\n1157\t0.036264\t2.410668\t2.615527\t1.519406\t0.678026\t0.71168\n1158\t0.036784\t2.409961\t2.615977\t1.516626\t0.677488\t0.711294\n1159\t0.037305\t2.409323\t2.616296\t1.513846\t0.676951\t0.710908\n1160\t0.037825\t2.408686\t2.616615\t1.511065\t0.676413\t0.710521\n1161\t0.038345\t2.408048\t2.616934\t1.508285\t0.675876\t0.710135\n1162\t0.038865\t2.40741\t2.617252\t1.505504\t0.675338\t0.709749\n1163\t0.039386\t2.406773\t2.617571\t1.502724\t0.6748\t0.709362\n1164\t0.039906\t2.406135\t2.61789\t1.499943\t0.674263\t0.708976\n1165\t0.040164\t2.405498\t2.618209\t1.497163\t0.673725\t0.70859\n1166\t0.04025\t2.40486\t2.618528\t1.494382\t0.673188\t0.708203\n1167\t0.040337\t2.404222\t2.618846\t1.491602\t0.67265\t0.707817\n1168\t0.040424\t2.403585\t2.619165\t1.488821\t0.672113\t0.707431\n1169\t0.04051\t2.402947\t2.619484\t1.486041\t0.671575\t0.707044\n1170\t0.040597\t2.40231\t2.619803\t1.48326\t0.671038\t0.706658\n1171\t0.040684\t2.401672\t2.620122\t1.48048\t0.6705\t0.706272\n1172\t0.040771\t2.401034\t2.62044\t1.4777\t0.669962\t0.705885\n1173\t0.040857\t2.400375\t2.62069\t1.474919\t0.669425\t0.705499\n1174\t0.040944\t2.399652\t2.620743\t1.472139\t0.668985\t0.705113\n1175\t0.041031\t2.398929\t2.620796\t1.469358\t0.668559\t0.704726\n1176\t0.041117\t2.398207\t2.620849\t1.466578\t0.668132\t0.70434\n1177\t0.041204\t2.397484\t2.620902\t1.463797\t0.667706\t0.703953\n1178\t0.041291\t2.396762\t2.620955\t1.461017\t0.66728\t0.703567\n1179\t0.041378\t2.396039\t2.621008\t1.458236\t0.666853\t0.703181\n1180\t0.041456\t2.395316\t2.621061\t1.455766\t0.666427\t0.702794\n1181\t0.041518\t2.394594\t2.621115\t1.453487\t0.666001\t0.702408\n1182\t0.041579\t2.393871\t2.621168\t1.451207\t0.665574\t0.702022\n1183\t0.04164\t2.393149\t2.621221\t1.448927\t0.665148\t0.701635\n1184\t0.041701\t2.392426\t2.621274\t1.446647\t0.664722\t0.701249\n1185\t0.041763\t2.391703\t2.621327\t1.444367\t0.664295\t0.700863\n1186\t0.041824\t2.390981\t2.62138\t1.442087\t0.663869\t0.700475\n1187\t0.041885\t2.390258\t2.621433\t1.439807\t0.663443\t0.700086\n1188\t0.041946\t2.389536\t2.621487\t1.437527\t0.663016\t0.699697\n1189\t0.042007\t2.388711\t2.621775\t1.435247\t0.66259\t0.699308\n1190\t0.042069\t2.387882\t2.622073\t1.432967\t0.662164\t0.698918\n1191\t0.04213\t2.387053\t2.62237\t1.430687\t0.661737\t0.698529\n1192\t0.042191\t2.386224\t2.622668\t1.428407\t0.661311\t0.69814\n1193\t0.042252\t2.385395\t2.622965\t1.426127\t0.660885\t0.697751\n1194\t0.042313\t2.384566\t2.623263\t1.423847\t0.660458\t0.697361\n1195\t0.042373\t2.383737\t2.623561\t1.421567\t0.660032\t0.696972\n1196\t0.042312\t2.382908\t2.623858\t1.419287\t0.659606\t0.696583\n1197\t0.042251\t2.38208\t2.624156\t1.417007\t0.659179\t0.696193\n1198\t0.04219\t2.381251\t2.624453\t1.414727\t0.658753\t0.695804\n1199\t0.042129\t2.380422\t2.624751\t1.412447\t0.658327\t0.695415\n1200\t0.042067\t2.379593\t2.625048\t1.410167\t0.6579\t0.695026\n1201\t0.042006\t2.378764\t2.625346\t1.407887\t0.657474\t0.694636\n1202\t0.041945\t2.377935\t2.625643\t1.405607\t0.657048\t0.694247\n1203\t0.041884\t2.377106\t2.625941\t1.403327\t0.656621\t0.693858\n1204\t0.041823\t2.376306\t2.625849\t1.401047\t0.656195\t0.693469\n1205\t0.041761\t2.375519\t2.625562\t1.398767\t0.655769\t0.693079\n1206\t0.0417\t2.374733\t2.625275\t1.396487\t0.655342\t0.69269\n1207\t0.041639\t2.373947\t2.624988\t1.394207\t0.654916\t0.692301\n1208\t0.041578\t2.37316\t2.624702\t1.391927\t0.654601\t0.691912\n1209\t0.041516\t2.372374\t2.624415\t1.389647\t0.654416\t0.691522\n1210\t0.041455\t2.371588\t2.624128\t1.387367\t0.65423\t0.691133\n1211\t0.041401\t2.370801\t2.623841\t1.385087\t0.654045\t0.690744\n1212\t0.04135\t2.370015\t2.623554\t1.382807\t0.65386\t0.690355\n1213\t0.041299\t2.369229\t2.623267\t1.380527\t0.653674\t0.689965\n1214\t0.041248\t2.368442\t2.62298\t1.378201\t0.653489\t0.689576\n1215\t0.041197\t2.367656\t2.622693\t1.375699\t0.653304\t0.689187\n1216\t0.041146\t2.366869\t2.622406\t1.373197\t0.653118\t0.688797\n1217\t0.041095\t2.366083\t2.622119\t1.370694\t0.652933\t0.688408\n1218\t0.041044\t2.365297\t2.621832\t1.368192\t0.652748\t0.688019\n1219\t0.040993\t2.36451\t2.621225\t1.365689\t0.652562\t0.68763\n1220\t0.040942\t2.363724\t2.620067\t1.363187\t0.652377\t0.68724\n1221\t0.040891\t2.362938\t2.618908\t1.360685\t0.652191\t0.687309\n1222\t0.04084\t2.362151\t2.61775\t1.358182\t0.652006\t0.687401\n1223\t0.040789\t2.361365\t2.616592\t1.35568\t0.651821\t0.687494\n1224\t0.040738\t2.360579\t2.615433\t1.353177\t0.651635\t0.687587\n1225\t0.040687\t2.359792\t2.614275\t1.350675\t0.65145\t0.687679\n1226\t0.040604\t2.359006\t2.613117\t1.348172\t0.651265\t0.687772\n1227\t0.040477\t2.35822\t2.611959\t1.34567\t0.651079\t0.687865\n1228\t0.040349\t2.357433\t2.6108\t1.343168\t0.650894\t0.687957\n1229\t0.040222\t2.356647\t2.609642\t1.340665\t0.650709\t0.68805\n1230\t0.040094\t2.35586\t2.608484\t1.338163\t0.650523\t0.688143\n1231\t0.039967\t2.355074\t2.607325\t1.33566\t0.650338\t0.688235\n1232\t0.039839\t2.354288\t2.606167\t1.333158\t0.650152\t0.688328\n1233\t0.039712\t2.353501\t2.605009\t1.330656\t0.649967\t0.688421\n1234\t0.039584\t2.352722\t2.603891\t1.328153\t0.649782\t0.688514\n1235\t0.039457\t2.352042\t2.603306\t1.325651\t0.649596\t0.688606\n1236\t0.039329\t2.351362\t2.602722\t1.323148\t0.649411\t0.688699\n1237\t0.039202\t2.350682\t2.602137\t1.320646\t0.649226\t0.688792\n1238\t0.039074\t2.350002\t2.601553\t1.318144\t0.64904\t0.688884\n1239\t0.038947\t2.349322\t2.600968\t1.315641\t0.648855\t0.688977\n1240\t0.038819\t2.348642\t2.600384\t1.313139\t0.64867\t0.68907\n1241\t0.038704\t2.347962\t2.599799\t1.310636\t0.648484\t0.689162\n1242\t0.038684\t2.347282\t2.599215\t1.308134\t0.648289\t0.689255\n1243\t0.038663\t2.346602\t2.598631\t1.305631\t0.6479\t0.689348\n1244\t0.038643\t2.345921\t2.598046\t1.303129\t0.64751\t0.68944\n1245\t0.038622\t2.345241\t2.597462\t1.300627\t0.647121\t0.689533\n1246\t0.038602\t2.344561\t2.596877\t1.298124\t0.646732\t0.689626\n1247\t0.038582\t2.343881\t2.596293\t1.295622\t0.646342\t0.689718\n1248\t0.038561\t2.343201\t2.595708\t1.293119\t0.645953\t0.689811\n1249\t0.038541\t2.342521\t2.595124\t1.291219\t0.645564\t0.689904\n1250\t0.03852\t2.341742\t2.594589\t1.289477\t0.645175\t0.689996\n1251\t0.0385\t2.340935\t2.594068\t1.287734\t0.644785\t0.690089\n1252\t0.03848\t2.340127\t2.593547\t1.285992\t0.644396\t0.690182\n1253\t0.038459\t2.33932\t2.593026\t1.284249\t0.644007\t0.690274\n1254\t0.038439\t2.338512\t2.592506\t1.282507\t0.643618\t0.690367\n1255\t0.038418\t2.337704\t2.591985\t1.280765\t0.643228\t0.690281\n1256\t0.038398\t2.336897\t2.591464\t1.279022\t0.642839\t0.69004\n1257\t0.038365\t2.336089\t2.590944\t1.27728\t0.64245\t0.689799\n1258\t0.038329\t2.335282\t2.590423\t1.275537\t0.642061\t0.689558\n1259\t0.038294\t2.334474\t2.589902\t1.273795\t0.641671\t0.689317\n1260\t0.038258\t2.333666\t2.589382\t1.272053\t0.641282\t0.689076\n1261\t0.038222\t2.332859\t2.588861\t1.27031\t0.640893\t0.688835\n1262\t0.038186\t2.332051\t2.58834\t1.268568\t0.640503\t0.688594\n1263\t0.038151\t2.331243\t2.587819\t1.266825\t0.640114\t0.688353\n1264\t0.038115\t2.330436\t2.587299\t1.265083\t0.639725\t0.688113\n1265\t0.038079\t2.329774\t2.586959\t1.26334\t0.639336\t0.687872\n1266\t0.038044\t2.329275\t2.586821\t1.261598\t0.638946\t0.687631\n1267\t0.038008\t2.328775\t2.586683\t1.259856\t0.638557\t0.68739\n1268\t0.037972\t2.328276\t2.586545\t1.258113\t0.638168\t0.687149\n1269\t0.037936\t2.327776\t2.586407\t1.256371\t0.637779\t0.686908\n1270\t0.037901\t2.327277\t2.586269\t1.254628\t0.637389\t0.686667\n1271\t0.037865\t2.326778\t2.586131\t1.252886\t0.637\t0.686426\n1272\t0.037914\t2.326278\t2.585992\t1.251144\t0.636611\t0.686185\n1273\t0.038042\t2.325779\t2.585854\t1.249401\t0.636222\t0.685944\n1274\t0.038169\t2.325279\t2.585716\t1.247659\t0.635832\t0.685703\n1275\t0.038297\t2.32478\t2.585578\t1.245916\t0.635443\t0.685462\n1276\t0.038424\t2.32428\t2.58544\t1.244174\t0.635054\t0.685221\n1277\t0.038552\t2.323781\t2.585302\t1.242431\t0.634723\t0.68498\n1278\t0.038679\t2.323281\t2.585164\t1.240689\t0.634427\t0.684739\n1279\t0.038807\t2.322782\t2.585025\t1.238947\t0.63413\t0.684498\n1280\t0.038935\t2.322256\t2.584912\t1.237204\t0.633834\t0.684257\n1281\t0.039062\t2.321608\t2.584912\t1.235462\t0.633537\t0.684016\n1282\t0.03919\t2.32096\t2.584912\t1.233719\t0.633241\t0.683775\n1283\t0.039317\t2.320312\t2.584912\t1.231816\t0.632944\t0.683534\n1284\t0.039445\t2.319664\t2.584912\t1.229647\t0.632647\t0.683293\n1285\t0.039572\t2.319015\t2.584912\t1.227478\t0.632351\t0.683052\n1286\t0.0397\t2.318367\t2.584912\t1.225309\t0.632054\t0.682811\n1287\t0.0399\t2.317719\t2.584912\t1.223141\t0.631758\t0.68257\n1288\t0.040354\t2.317071\t2.584912\t1.220972\t0.631461\t0.682329\n1289\t0.040808\t2.316422\t2.584912\t1.218803\t0.631164\t0.682093\n1290\t0.041262\t2.315774\t2.584912\t1.216634\t0.630868\t0.681889\n1291\t0.041716\t2.315126\t2.584912\t1.214466\t0.630571\t0.681685\n1292\t0.04217\t2.314478\t2.584912\t1.212297\t0.630275\t0.681481\n1293\t0.042624\t2.31383\t2.584912\t1.210128\t0.629978\t0.681277\n1294\t0.043078\t2.313181\t2.584912\t1.207959\t0.629682\t0.681073\n1295\t0.043532\t2.312533\t2.584912\t1.205791\t0.629385\t0.680869\n1296\t0.043986\t2.311838\t2.584996\t1.203622\t0.629088\t0.680665\n1297\t0.04444\t2.311137\t2.585091\t1.201453\t0.628792\t0.680461\n1298\t0.044894\t2.310436\t2.585187\t1.199284\t0.628495\t0.680258\n1299\t0.045348\t2.309734\t2.585282\t1.197116\t0.628199\t0.680054\n1300\t0.045802\t2.309033\t2.585378\t1.194947\t0.627902\t0.67985\n1301\t0.046256\t2.308332\t2.585474\t1.192778\t0.627605\t0.679646\n1302\t0.04671\t2.30763\t2.585569\t1.190609\t0.627309\t0.679442\n1303\t0.047503\t2.306929\t2.585665\t1.18844\t0.627012\t0.679238\n1304\t0.048325\t2.306227\t2.585761\t1.186272\t0.626716\t0.679034\n1305\t0.049146\t2.305526\t2.585856\t1.184103\t0.626419\t0.67883\n1306\t0.049967\t2.304825\t2.585952\t1.181934\t0.626123\t0.678626\n1307\t0.050788\t2.304123\t2.586048\t1.179765\t0.625826\t0.678422\n1308\t0.05161\t2.303422\t2.586143\t1.177597\t0.625529\t0.678219\n1309\t0.052431\t2.302721\t2.586239\t1.175428\t0.625233\t0.678015\n1310\t0.053252\t2.302019\t2.586334\t1.173259\t0.624936\t0.677811\n1311\t0.054074\t2.301441\t2.586726\t1.17109\t0.624652\t0.677607\n1312\t0.054895\t2.300952\t2.587332\t1.168922\t0.624411\t0.677403\n1313\t0.055716\t2.300464\t2.587937\t1.166753\t0.62417\t0.677199\n1314\t0.056537\t2.299975\t2.588543\t1.164584\t0.623929\t0.676995\n1315\t0.057359\t2.299486\t2.589149\t1.162415\t0.623688\t0.676791\n1316\t0.05818\t2.298997\t2.589755\t1.160247\t0.623447\t0.676587\n1317\t0.059001\t2.298508\t2.59036\t1.158078\t0.623206\t0.676383\n1318\t0.060089\t2.29802\t2.590966\t1.156374\t0.622965\t0.67618\n1319\t0.061336\t2.297531\t2.591572\t1.154687\t0.622724\t0.675976\n1320\t0.062583\t2.297042\t2.592177\t1.153\t0.622483\t0.675772\n1321\t0.06383\t2.296553\t2.592783\t1.151313\t0.622242\t0.675568\n1322\t0.065077\t2.296064\t2.593389\t1.149627\t0.622001\t0.675364\n1323\t0.066324\t2.295575\t2.593994\t1.14794\t0.62176\t0.67516\n1324\t0.067571\t2.295087\t2.5946\t1.146253\t0.621519\t0.67493\n1325\t0.068818\t2.294598\t2.595206\t1.144566\t0.621278\t0.674689\n1326\t0.070065\t2.294115\t2.595851\t1.142879\t0.621037\t0.674448\n1327\t0.071312\t2.293647\t2.596594\t1.141193\t0.620796\t0.674207\n1328\t0.072559\t2.29318\t2.597338\t1.139506\t0.620555\t0.673966\n1329\t0.073806\t2.292712\t2.598082\t1.137819\t0.620314\t0.673725\n1330\t0.075053\t2.292245\t2.598826\t1.136132\t0.620073\t0.673484\n1331\t0.076299\t2.291777\t2.59957\t1.134445\t0.619832\t0.673243\n1332\t0.07779\t2.29131\t2.600314\t1.132758\t0.619591\t0.673002\n1333\t0.079375\t2.290842\t2.601058\t1.131072\t0.619351\t0.672761\n1334\t0.08096\t2.290374\t2.601801\t1.129385\t0.61911\t0.67252\n1335\t0.082545\t2.289907\t2.602545\t1.127698\t0.618869\t0.672279\n1336\t0.08413\t2.289439\t2.603289\t1.126011\t0.618628\t0.672038\n1337\t0.085715\t2.288972\t2.604033\t1.124324\t0.618387\t0.671797\n1338\t0.0873\t2.288504\t2.604777\t1.122638\t0.618146\t0.671556\n1339\t0.088885\t2.288037\t2.605521\t1.120951\t0.617905\t0.671315\n1340\t0.09047\t2.287569\t2.606265\t1.119264\t0.617664\t0.671074\n1341\t0.092055\t2.287102\t2.607008\t1.117577\t0.617423\t0.670833\n1342\t0.09364\t2.286634\t2.60793\t1.11589\t0.617182\t0.670592\n1343\t0.095225\t2.286166\t2.608855\t1.114204\t0.616941\t0.670351\n1344\t0.096763\t2.285699\t2.609779\t1.112517\t0.6167\t0.670111\n1345\t0.098118\t2.285231\t2.610704\t1.11083\t0.616459\t0.66987\n1346\t0.099473\t2.284764\t2.611628\t1.109143\t0.616173\t0.669629\n1347\t0.100829\t2.284296\t2.612553\t1.107456\t0.615876\t0.669388\n1348\t0.102184\t2.283829\t2.613477\t1.105769\t0.61558\t0.669147\n1349\t0.103539\t2.283361\t2.614402\t1.104083\t0.615283\t0.668906\n1350\t0.104894\t2.282893\t2.615326\t1.102396\t0.614987\t0.668665\n1351\t0.106249\t2.282426\t2.616251\t1.100709\t0.61469\t0.668424\n1352\t0.107605\t2.281958\t2.617175\t1.099002\t0.614393\t0.668183\n1353\t0.10896\t2.281491\t2.6181\t1.097278\t0.614097\t0.667942\n1354\t0.110315\t2.281023\t2.619024\t1.095554\t0.6138\t0.667701\n1355\t0.11167\t2.280556\t2.619949\t1.09383\t0.613504\t0.66746\n1356\t0.113025\t2.280088\t2.620873\t1.092106\t0.613207\t0.667219\n1357\t0.114381\t2.279708\t2.622082\t1.090382\t0.612911\t0.666978\n1358\t0.116059\t2.279368\t2.623421\t1.088659\t0.612614\t0.666769\n1359\t0.117793\t2.279028\t2.62476\t1.086935\t0.612317\t0.66664\n1360\t0.119528\t2.278688\t2.626099\t1.085211\t0.612021\t0.66651\n1361\t0.121262\t2.278348\t2.627438\t1.083487\t0.611724\t0.66638\n1362\t0.122997\t2.278008\t2.628777\t1.081763\t0.611428\t0.66625\n1363\t0.124731\t2.277668\t2.630116\t1.080039\t0.611131\t0.666121\n1364\t0.126466\t2.277328\t2.631455\t1.078315\t0.610835\t0.665991\n1365\t0.1282\t2.276988\t2.632794\t1.076591\t0.610538\t0.665861\n1366\t0.129935\t2.276648\t2.634132\t1.074867\t0.610241\t0.665731\n1367\t0.13167\t2.276307\t2.635471\t1.073144\t0.609945\t0.665602\n1368\t0.133404\t2.275967\t2.63681\t1.07142\t0.609648\t0.665472\n1369\t0.136488\t2.275627\t2.638149\t1.069696\t0.609352\t0.665342\n1370\t0.139782\t2.275287\t2.639488\t1.067972\t0.609055\t0.665212\n1371\t0.143077\t2.274947\t2.640827\t1.066248\t0.608758\t0.665083\n1372\t0.146371\t2.274762\t2.642822\t1.064524\t0.608462\t0.664953\n1373\t0.149665\t2.274821\t2.645851\t1.0628\t0.608165\t0.664823\n1374\t0.15296\t2.274879\t2.64888\t1.061076\t0.607869\t0.664693\n1375\t0.156904\t2.274938\t2.651909\t1.059353\t0.607572\t0.664564\n1376\t0.161636\t2.274996\t2.654938\t1.057629\t0.607276\t0.664434\n1377\t0.166369\t2.275055\t2.657967\t1.055905\t0.606979\t0.664304\n1378\t0.171101\t2.275114\t2.660996\t1.054181\t0.606682\t0.664174\n1379\t0.175833\t2.275172\t2.664025\t1.052457\t0.606386\t0.664045\n1380\t0.180565\t2.275231\t2.667054\t1.050733\t0.606082\t0.663915\n1381\t0.19244\t2.27529\t2.670083\t1.049009\t0.605767\t0.663785\n1382\t0.205204\t2.275348\t2.673112\t1.047285\t0.605452\t0.663655\n1383\t0.211768\t2.275407\t2.676141\t1.045561\t0.605137\t0.663526\n1384\t0.218058\t2.275465\t2.679286\t1.043838\t0.604821\t0.663396\n1385\t0.224348\t2.275524\t2.686787\t1.042114\t0.604506\t0.663266\n1386\t0.236666\t2.275583\t2.694287\t1.040443\t0.604191\t0.663136\n1387\t0.251961\t2.275738\t2.701788\t1.039108\t0.603876\t0.663007\n1388\t0.264353\t2.275972\t2.709288\t1.037774\t0.603561\t0.662877\n1389\t0.286325\t2.276205\t2.716789\t1.036439\t0.603246\t0.662747\n1390\t0.295374\t2.276439\t2.724289\t1.035104\t0.602931\t0.662617\n1391\t0.304422\t2.276673\t2.732984\t1.03377\t0.602616\t0.662488\n1392\t0.321093\t2.276906\t2.742713\t1.032435\t0.6023\t0.662358\n1393\t0.353026\t2.27714\t2.752441\t1.0311\t0.601985\t0.662342\n1394\t0.37652\t2.277373\t2.76217\t1.029766\t0.60167\t0.662342\n1395\t0.395208\t2.277607\t2.77387\t1.028431\t0.601355\t0.662342\n1396\t0.410951\t2.277841\t2.788067\t1.027097\t0.60104\t0.662342\n1397\t0.422102\t2.278074\t2.802265\t1.025762\t0.600725\t0.662342\n1398\t0.433254\t2.278308\t2.81225\t1.024427\t0.60041\t0.662342\n1399\t0.472582\t2.278542\t2.820063\t1.023093\t0.600095\t0.662342\n1400\t0.52\t2.278775\t2.827876\t1.021758\t0.59978\t0.662342\n1401\t0.544279\t2.279009\t2.835689\t1.020423\t0.599464\t0.662342\n1402\t0.535005\t2.279242\t2.843502\t1.019089\t0.599149\t0.662342\n1403\t0.563781\t2.27983\t2.850739\t1.017754\t0.598834\t0.662342\n1404\t0.584661\t2.28051\t2.85732\t1.01642\t0.598519\t0.662342\n1405\t0.60028\t2.28119\t2.863902\t1.015085\t0.598204\t0.662342\n1406\t0.616118\t2.28187\t2.870483\t1.01375\t0.597889\t0.662342\n1407\t0.63243\t2.28255\t2.877065\t1.012416\t0.597574\t0.662342\n1408\t0.661912\t2.28323\t2.883646\t1.011081\t0.597259\t0.662342\n1409\t0.681384\t2.28391\t2.890228\t1.009746\t0.596943\t0.662342\n1410\t0.705194\t2.28459\t2.901174\t1.008412\t0.596628\t0.662342\n1411\t0.720839\t2.285271\t2.912961\t1.007077\t0.596313\t0.662342\n1412\t0.732439\t2.285951\t2.924503\t1.005743\t0.595998\t0.662342\n1413\t0.760611\t2.286631\t2.932004\t1.004408\t0.595683\t0.662342\n1414\t0.777271\t2.287311\t2.939506\t1.003073\t0.595368\t0.662342\n1415\t0.79318\t2.287991\t2.947008\t1.001739\t0.595162\t0.662342\n1416\t0.809404\t2.288671\t2.95451\t1.000404\t0.594958\t0.662342\n1417\t0.821148\t2.289351\t2.962012\t0.99907\t0.594754\t0.662342\n1418\t0.83788\t2.289926\t2.969118\t0.997735\t0.59455\t0.662342\n1419\t0.854374\t2.290394\t2.975028\t0.9964\t0.594346\t0.662342\n1420\t0.865947\t2.290861\t2.980938\t0.995066\t0.594142\t0.662342\n1421\t0.877521\t2.291329\t2.986848\t0.993691\t0.593938\t0.662342\n1422\t0.889794\t2.291796\t2.992758\t0.992301\t0.593734\t0.662342\n1423\t0.902584\t2.292264\t2.99808\t0.99091\t0.59353\t0.662342\n1424\t0.914097\t2.292732\t3.001259\t0.98952\t0.593327\t0.662342\n1425\t0.921477\t2.293199\t3.004437\t0.98813\t0.593123\t0.662342\n1426\t0.928858\t2.293667\t3.007616\t0.98674\t0.592919\t0.662342\n1427\t0.936279\t2.294134\t3.010795\t0.98535\t0.592715\t0.66223\n1428\t0.943924\t2.294602\t3.013973\t0.983959\t0.592511\t0.661989\n1429\t0.951568\t2.295069\t3.017152\t0.982569\t0.592307\t0.661748\n1430\t0.959213\t2.295537\t3.019908\t0.981179\t0.592103\t0.661507\n1431\t0.968235\t2.296005\t3.021788\t0.979789\t0.591899\t0.661266\n1432\t0.977594\t2.296472\t3.023668\t0.978398\t0.591695\t0.661025\n1433\t0.985955\t2.296835\t3.025547\t0.977008\t0.591491\t0.660784\n1434\t0.990228\t2.296772\t3.027427\t0.975618\t0.591288\t0.660543\n1435\t0.994502\t2.296708\t3.029307\t0.974228\t0.591084\t0.660302\n1436\t0.998776\t2.296644\t3.031187\t0.972837\t0.59088\t0.660061\n1437\t1.00305\t2.29658\t3.033066\t0.971447\t0.590676\t0.65982\n1438\t1.007324\t2.296517\t3.034946\t0.970057\t0.590472\t0.659579\n1439\t1.01076\t2.296453\t3.036826\t0.968667\t0.590268\t0.659338\n1440\t1.013712\t2.296389\t3.038706\t0.967277\t0.590064\t0.659097\n1441\t1.016663\t2.296325\t3.040586\t0.965886\t0.58986\t0.658856\n1442\t1.019614\t2.296262\t3.042465\t0.964496\t0.589656\t0.658615\n1443\t1.022566\t2.296198\t3.044345\t0.963106\t0.589452\t0.658375\n1444\t1.025517\t2.296134\t3.046225\t0.961716\t0.589249\t0.658134\n1445\t1.028469\t2.29607\t3.048105\t0.960325\t0.589045\t0.657893\n1446\t1.03142\t2.296007\t3.048721\t0.958935\t0.588841\t0.657652\n1447\t1.033166\t2.295943\t3.048743\t0.957545\t0.588637\t0.657411\n1448\t1.033139\t2.295879\t3.048764\t0.956155\t0.588433\t0.65717\n1449\t1.033112\t2.295653\t3.048785\t0.954765\t0.588177\t0.656929\n1450\t1.033085\t2.295409\t3.048806\t0.953374\t0.58788\t0.656688\n1451\t1.033059\t2.295164\t3.048828\t0.951984\t0.587584\t0.656447\n1452\t1.033032\t2.29492\t3.048849\t0.950594\t0.587287\t0.656206\n1453\t1.033005\t2.294675\t3.04887\t0.949204\t0.58699\t0.655965\n1454\t1.032978\t2.294431\t3.048891\t0.947813\t0.586694\t0.655724\n1455\t1.032951\t2.294187\t3.048913\t0.946435\t0.586397\t0.655483\n1456\t1.032924\t2.293942\t3.048934\t0.945081\t0.586101\t0.655242\n1457\t1.032898\t2.293698\t3.048955\t0.943728\t0.585804\t0.655001\n1458\t1.032871\t2.293453\t3.048976\t0.942375\t0.585507\t0.65476\n1459\t1.032844\t2.293209\t3.048998\t0.941022\t0.585211\t0.654519\n1460\t1.03254\t2.292965\t3.049019\t0.939669\t0.584914\t0.654278\n1461\t1.028923\t2.29272\t3.04816\t0.938316\t0.584618\t0.654041\n1462\t1.025305\t2.292476\t3.045876\t0.936962\t0.584321\t0.653874\n1463\t1.021687\t2.292231\t3.043591\t0.935609\t0.584025\t0.653707\n1464\t1.01807\t2.291738\t3.041306\t0.934256\t0.583728\t0.65354\n1465\t1.014452\t2.291079\t3.039022\t0.932903\t0.583431\t0.653373\n1466\t1.010834\t2.29042\t3.036737\t0.93155\t0.583135\t0.653207\n1467\t1.002847\t2.289762\t3.034453\t0.930197\t0.582838\t0.65304\n1468\t0.993892\t2.289103\t3.032168\t0.928844\t0.582542\t0.652873\n1469\t0.985476\t2.288444\t3.029883\t0.92749\t0.582245\t0.652706\n1470\t0.979326\t2.287785\t3.027599\t0.926137\t0.581948\t0.652539\n1471\t0.973175\t2.287126\t3.025314\t0.924784\t0.581652\t0.652372\n1472\t0.967025\t2.286467\t3.02303\t0.923431\t0.581355\t0.652206\n1473\t0.960875\t2.285809\t3.020745\t0.922078\t0.581059\t0.652039\n1474\t0.95159\t2.28515\t3.018461\t0.920725\t0.580762\t0.651872\n1475\t0.941817\t2.284491\t3.015428\t0.919371\t0.580466\t0.651705\n1476\t0.932988\t2.283832\t3.011566\t0.918018\t0.580169\t0.651538\n1477\t0.924939\t2.283173\t3.007704\t0.916665\t0.579872\t0.651372\n1478\t0.916556\t2.282514\t3.003842\t0.915312\t0.579576\t0.651205\n1479\t0.905063\t2.281904\t2.99998\t0.913959\t0.579279\t0.651038\n1480\t0.893613\t2.281404\t2.996118\t0.912606\t0.578983\t0.650871\n1481\t0.882762\t2.280905\t2.992256\t0.911252\t0.578686\t0.650704\n1482\t0.871911\t2.280405\t2.988394\t0.909899\t0.578389\t0.650537\n1483\t0.86106\t2.279906\t2.984533\t0.908546\t0.578093\t0.650371\n1484\t0.861266\t2.279406\t2.980671\t0.907193\t0.577796\t0.650204\n1485\t0.85893\t2.278907\t2.976809\t0.90584\t0.5775\t0.650037\n1486\t0.840385\t2.278408\t2.972983\t0.904487\t0.577203\t0.64987\n1487\t0.828105\t2.277908\t2.969224\t0.903134\t0.576907\t0.649703\n1488\t0.81915\t2.277409\t2.965465\t0.90178\t0.57661\t0.649536\n1489\t0.810498\t2.276909\t2.961706\t0.900427\t0.576313\t0.64937\n1490\t0.802077\t2.27641\t2.957947\t0.899273\t0.576017\t0.649203\n1491\t0.793657\t2.27591\t2.954188\t0.898142\t0.57572\t0.649036\n1492\t0.768816\t2.275411\t2.950429\t0.897011\t0.575424\t0.648869\n1493\t0.761177\t2.274911\t2.94667\t0.895881\t0.575127\t0.648702\n1494\t0.753735\t2.274411\t2.942911\t0.89475\t0.57483\t0.648535\n1495\t0.746293\t2.273603\t2.939152\t0.893619\t0.574534\t0.648369\n1496\t0.73995\t2.272795\t2.935622\t0.892489\t0.574237\t0.648308\n1497\t0.733651\t2.271988\t2.932237\t0.891358\t0.573941\t0.648308\n1498\t0.727352\t2.27118\t2.928852\t0.890227\t0.573644\t0.648308\n1499\t0.721053\t2.270373\t2.925467\t0.889096\t0.573348\t0.648308\n1500\t0.712875\t2.269565\t2.922082\t0.887966\t0.573051\t0.648308\n1501\t0.704498\t2.268757\t2.918697\t0.886835\t0.572754\t0.648308\n1502\t0.696122\t2.26795\t2.915312\t0.885704\t0.572458\t0.648308\n1503\t0.68409\t2.267142\t2.911926\t0.884574\t0.572161\t0.648308\n1504\t0.668194\t2.266335\t2.908541\t0.883443\t0.571865\t0.648308\n1505\t0.660427\t2.265527\t2.905156\t0.882312\t0.571568\t0.648308\n1506\t0.653856\t2.264719\t2.901322\t0.881181\t0.571271\t0.648308\n1507\t0.647284\t2.263912\t2.897425\t0.880051\t0.570975\t0.648308\n1508\t0.64038\t2.263104\t2.893528\t0.87892\t0.570678\t0.648308\n1509\t0.633136\t2.262296\t2.889631\t0.877789\t0.570382\t0.648308\n1510\t0.625892\t2.261451\t2.885734\t0.876659\t0.570085\t0.648308\n1511\t0.618064\t2.260591\t2.881837\t0.875528\t0.569789\t0.648308\n1512\t0.606692\t2.25973\t2.87794\t0.874397\t0.569492\t0.648308\n1513\t0.596649\t2.258869\t2.874044\t0.873266\t0.569195\t0.648308\n1514\t0.591072\t2.258008\t2.87012\t0.872136\t0.568899\t0.648308\n1515\t0.585495\t2.257148\t2.865872\t0.871005\t0.568602\t0.648308\n1516\t0.579918\t2.256287\t2.861624\t0.869874\t0.568306\t0.648308\n1517\t0.573738\t2.255426\t2.857376\t0.868743\t0.568009\t0.648308\n1518\t0.56736\t2.254565\t2.853128\t0.867613\t0.567849\t0.648308\n1519\t0.560981\t2.253705\t2.84888\t0.866482\t0.567738\t0.648308\n1520\t0.552996\t2.252844\t2.844632\t0.865351\t0.567627\t0.648308\n1521\t0.54404\t2.251983\t2.840384\t0.864221\t0.567515\t0.648308\n1522\t0.535546\t2.251122\t2.836137\t0.86309\t0.567404\t0.648308\n1523\t0.529027\t2.250262\t2.831889\t0.861959\t0.567293\t0.648308\n1524\t0.522508\t2.249401\t2.827641\t0.860704\t0.567182\t0.648308\n1525\t0.51599\t2.248588\t2.824144\t0.859314\t0.567071\t0.648308\n1526\t0.509529\t2.247844\t2.821735\t0.857923\t0.566959\t0.648308\n1527\t0.503072\t2.2471\t2.819326\t0.856533\t0.566848\t0.648308\n1528\t0.496614\t2.246356\t2.816918\t0.855143\t0.566737\t0.648308\n1529\t0.489848\t2.245612\t2.814509\t0.853753\t0.566626\t0.648308\n1530\t0.483058\t2.244869\t2.8121\t0.852363\t0.566514\t0.648287\n1531\t0.476478\t2.244125\t2.809692\t0.850972\t0.566403\t0.648195\n1532\t0.471088\t2.243381\t2.807283\t0.849582\t0.566292\t0.648102\n1533\t0.465697\t2.242637\t2.804874\t0.848192\t0.566181\t0.648009\n1534\t0.460307\t2.241893\t2.802466\t0.846802\t0.56607\t0.647917\n1535\t0.455121\t2.241149\t2.800057\t0.845411\t0.565958\t0.647824\n1536\t0.450035\t2.240405\t2.797648\t0.844021\t0.565847\t0.647731\n1537\t0.444949\t2.239662\t2.79524\t0.842631\t0.565736\t0.647639\n1538\t0.439863\t2.238918\t2.792831\t0.841241\t0.565625\t0.647546\n1539\t0.433906\t2.238174\t2.790422\t0.839851\t0.565514\t0.647453\n1540\t0.426158\t2.237438\t2.788011\t0.83846\t0.565402\t0.647361\n1541\t0.418411\t2.236769\t2.785577\t0.83707\t0.565291\t0.647268\n1542\t0.413577\t2.236099\t2.783144\t0.83568\t0.56518\t0.647175\n1543\t0.409879\t2.23543\t2.78071\t0.83429\t0.565069\t0.647083\n1544\t0.406181\t2.23476\t2.778277\t0.832899\t0.564957\t0.64699\n1545\t0.402483\t2.234091\t2.775843\t0.831509\t0.564846\t0.646897\n1546\t0.398785\t2.233421\t2.77341\t0.830119\t0.564735\t0.646804\n1547\t0.394992\t2.232752\t2.770977\t0.828729\t0.564624\t0.646712\n1548\t0.390686\t2.232082\t2.768543\t0.827338\t0.564513\t0.646619\n1549\t0.38638\t2.231413\t2.76611\t0.825948\t0.564401\t0.646526\n1550\t0.382074\t2.230743\t2.763676\t0.824558\t0.56429\t0.646434\n1551\t0.377768\t2.230074\t2.761243\t0.823168\t0.564179\t0.646341\n1552\t0.373549\t2.229405\t2.758809\t0.821778\t0.56399\t0.646248\n1553\t0.369545\t2.228735\t2.756376\t0.820387\t0.563638\t0.646156\n1554\t0.36554\t2.228066\t2.753942\t0.818997\t0.563286\t0.646063\n1555\t0.361535\t2.227396\t2.751509\t0.817607\t0.562933\t0.64597\n1556\t0.357531\t2.226777\t2.749541\t0.816217\t0.562581\t0.645878\n1557\t0.353721\t2.226169\t2.747682\t0.814826\t0.562229\t0.645785\n1558\t0.350177\t2.225562\t2.745822\t0.813462\t0.561877\t0.645692\n1559\t0.346634\t2.224954\t2.743963\t0.812461\t0.561525\t0.6456\n1560\t0.343091\t2.224347\t2.742103\t0.81146\t0.561172\t0.645507\n1561\t0.339547\t2.223739\t2.740243\t0.810459\t0.56082\t0.645414\n1562\t0.336004\t2.223131\t2.738384\t0.809458\t0.560468\t0.645322\n1563\t0.332398\t2.222524\t2.736524\t0.808457\t0.560116\t0.645229\n1564\t0.328595\t2.221916\t2.734664\t0.807456\t0.559764\t0.645136\n1565\t0.324791\t2.221309\t2.732805\t0.806455\t0.559411\t0.644864\n1566\t0.320988\t2.220701\t2.730945\t0.805454\t0.559059\t0.644549\n1567\t0.317184\t2.220093\t2.729085\t0.804453\t0.558707\t0.644233\n1568\t0.31338\t2.219486\t2.727226\t0.803452\t0.558355\t0.643918\n1569\t0.309982\t2.218878\t2.725366\t0.802451\t0.558003\t0.643603\n1570\t0.306952\t2.218271\t2.723506\t0.80145\t0.55765\t0.643288\n1571\t0.303921\t2.217717\t2.721827\t0.800449\t0.557298\t0.642973\n1572\t0.300891\t2.217214\t2.720318\t0.799448\t0.556946\t0.642658\n1573\t0.297861\t2.216711\t2.718809\t0.798447\t0.556594\t0.642343\n1574\t0.294831\t2.216208\t2.7173\t0.797446\t0.556242\t0.642028\n1575\t0.291801\t2.215705\t2.715791\t0.796445\t0.555889\t0.641712\n1576\t0.289726\t2.215202\t2.714282\t0.795444\t0.555537\t0.641397\n1577\t0.288014\t2.214699\t2.712773\t0.794443\t0.555185\t0.641082\n1578\t0.286303\t2.214196\t2.711264\t0.793442\t0.554833\t0.640767\n1579\t0.284591\t2.213693\t2.709756\t0.792441\t0.554481\t0.640452\n1580\t0.282879\t2.21319\t2.708247\t0.79144\t0.554129\t0.640137\n1581\t0.281168\t2.212687\t2.706738\t0.79044\t0.553776\t0.639822\n1582\t0.279456\t2.212185\t2.705229\t0.789439\t0.553424\t0.639507\n1583\t0.277744\t2.211682\t2.70372\t0.788438\t0.553072\t0.639192\n1584\t0.275857\t2.211179\t2.702211\t0.787437\t0.55272\t0.638876\n1585\t0.273787\t2.210676\t2.700702\t0.786436\t0.552368\t0.638561\n1586\t0.271717\t2.210116\t2.699269\t0.785435\t0.552015\t0.638246\n1587\t0.269648\t2.209507\t2.69811\t0.784434\t0.551933\t0.637931\n1588\t0.267578\t2.208898\t2.696952\t0.783433\t0.551877\t0.637616\n1589\t0.265508\t2.20829\t2.695794\t0.782432\t0.551821\t0.637301\n1590\t0.263439\t2.207681\t2.694635\t0.781431\t0.551766\t0.636986\n1591\t0.261369\t2.207072\t2.693477\t0.78043\t0.55171\t0.636671\n1592\t0.259299\t2.206463\t2.692319\t0.779429\t0.551655\t0.636355\n1593\t0.257372\t2.205855\t2.691161\t0.778609\t0.551599\t0.63604\n1594\t0.255844\t2.205246\t2.690002\t0.777886\t0.551543\t0.635725\n1595\t0.254317\t2.204637\t2.688844\t0.777163\t0.551488\t0.63541\n1596\t0.252789\t2.204029\t2.687686\t0.77644\t0.551432\t0.635095\n1597\t0.251262\t2.20342\t2.686527\t0.775717\t0.551377\t0.63478\n1598\t0.249734\t2.202811\t2.685369\t0.774995\t0.551321\t0.634465\n1599\t0.248207\t2.202202\t2.684211\t0.774272\t0.551265\t0.634274\n1600\t0.246679\t2.201594\t2.683053\t0.773549\t0.55121\t0.634274\n1601\t0.245151\t2.200985\t2.681894\t0.772826\t0.551154\t0.634274\n1602\t0.243624\t2.200379\t2.680863\t0.772103\t0.551099\t0.634274\n1603\t0.242096\t2.199773\t2.679843\t0.77138\t0.551043\t0.634274\n1604\t0.240569\t2.199167\t2.678823\t0.770657\t0.550987\t0.634274\n1605\t0.239041\t2.198562\t2.677802\t0.769934\t0.550932\t0.634274\n1606\t0.237531\t2.197956\t2.676782\t0.769211\t0.550876\t0.634274\n1607\t0.236336\t2.19735\t2.675762\t0.768488\t0.550821\t0.634274\n1608\t0.235141\t2.196745\t2.674742\t0.767765\t0.550765\t0.634274\n1609\t0.233946\t2.196139\t2.673722\t0.767042\t0.550709\t0.634274\n1610\t0.232751\t2.195533\t2.672702\t0.766319\t0.550654\t0.634274\n1611\t0.231556\t2.194927\t2.671682\t0.765597\t0.550598\t0.634274\n1612\t0.230361\t2.194322\t2.670661\t0.764874\t0.550542\t0.634274\n1613\t0.229166\t2.193716\t2.669641\t0.764151\t0.550487\t0.634274\n1614\t0.227971\t2.19311\t2.668621\t0.763428\t0.550431\t0.634274\n1615\t0.226776\t2.192505\t2.667601\t0.762705\t0.550376\t0.634274\n1616\t0.225581\t2.191899\t2.666581\t0.761982\t0.55032\t0.634274\n1617\t0.224386\t2.191333\t2.665706\t0.761259\t0.550264\t0.634274\n1618\t0.223191\t2.190791\t2.664919\t0.760536\t0.550209\t0.634274\n1619\t0.221997\t2.190249\t2.664133\t0.759813\t0.550153\t0.634274\n1620\t0.220802\t2.189707\t2.663347\t0.75909\t0.550098\t0.634274\n1621\t0.219795\t2.189165\t2.66256\t0.758367\t0.549877\t0.634274\n1622\t0.219019\t2.188623\t2.661774\t0.757644\t0.549488\t0.634274\n1623\t0.218244\t2.188081\t2.660988\t0.756922\t0.549098\t0.634274\n1624\t0.217469\t2.187539\t2.660201\t0.756199\t0.548709\t0.634274\n1625\t0.216693\t2.186997\t2.659415\t0.755476\t0.54832\t0.634274\n1626\t0.215918\t2.186455\t2.658628\t0.754753\t0.547931\t0.634274\n1627\t0.215142\t2.185913\t2.657842\t0.753942\t0.547541\t0.634274\n1628\t0.214367\t2.185371\t2.657056\t0.752848\t0.547152\t0.634274\n1629\t0.213592\t2.184829\t2.656269\t0.751755\t0.546763\t0.634274\n1630\t0.212816\t2.184287\t2.655483\t0.750661\t0.546374\t0.634274\n1631\t0.212041\t2.183745\t2.654697\t0.749567\t0.545984\t0.634274\n1632\t0.211266\t2.183269\t2.654088\t0.748474\t0.545595\t0.634274\n1633\t0.21049\t2.182928\t2.653855\t0.74738\t0.545206\t0.634274\n1634\t0.209715\t2.182588\t2.653621\t0.746286\t0.544817\t0.634274\n1635\t0.20894\t2.182248\t2.653387\t0.745193\t0.544427\t0.634274\n1636\t0.208189\t2.181908\t2.653153\t0.744099\t0.544038\t0.634274\n1637\t0.207577\t2.181568\t2.65292\t0.743005\t0.543649\t0.634274\n1638\t0.206964\t2.181228\t2.652686\t0.741912\t0.543259\t0.634274\n1639\t0.206352\t2.180888\t2.652452\t0.740818\t0.54287\t0.634274\n1640\t0.20574\t2.180548\t2.652218\t0.739724\t0.542481\t0.634274\n1641\t0.205128\t2.180208\t2.651984\t0.738631\t0.542092\t0.634274\n1642\t0.204516\t2.179868\t2.651751\t0.737537\t0.541702\t0.634274\n1643\t0.203904\t2.179528\t2.651517\t0.736443\t0.541313\t0.634274\n1644\t0.203292\t2.179188\t2.651283\t0.73535\t0.540924\t0.634274\n1645\t0.202679\t2.178848\t2.651049\t0.734256\t0.540535\t0.634274\n1646\t0.202067\t2.178508\t2.650816\t0.733163\t0.540145\t0.634274\n1647\t0.201455\t2.178165\t2.650594\t0.732069\t0.539756\t0.634274\n1648\t0.200843\t2.177719\t2.650881\t0.730975\t0.539367\t0.634274\n1649\t0.200231\t2.177273\t2.651168\t0.729882\t0.538978\t0.634274\n1650\t0.199619\t2.176826\t2.651455\t0.728788\t0.538588\t0.634274\n1651\t0.199007\t2.17638\t2.651742\t0.727694\t0.538199\t0.634274\n1652\t0.198468\t2.175934\t2.652029\t0.726601\t0.53781\t0.634274\n1653\t0.197943\t2.175487\t2.652316\t0.725507\t0.537421\t0.634274\n1654\t0.197418\t2.175041\t2.652603\t0.724413\t0.537031\t0.634274\n1655\t0.196892\t2.174595\t2.65289\t0.72332\t0.536667\t0.634274\n1656\t0.196367\t2.174148\t2.653177\t0.722226\t0.536586\t0.634274\n1657\t0.195841\t2.173702\t2.653464\t0.721132\t0.536506\t0.634274\n1658\t0.195316\t2.173256\t2.653751\t0.720039\t0.536425\t0.634274\n1659\t0.19479\t2.172809\t2.654037\t0.718945\t0.536345\t0.634274\n1660\t0.194265\t2.172363\t2.654324\t0.717851\t0.536264\t0.634274\n1661\t0.19374\t2.171917\t2.654611\t0.716758\t0.536184\t0.634274\n1662\t0.193214\t2.171471\t2.654898\t0.715827\t0.536103\t0.634274\n1663\t0.192689\t2.171287\t2.655525\t0.714932\t0.536023\t0.634274\n1664\t0.192163\t2.171202\t2.656279\t0.714036\t0.535942\t0.634274\n1665\t0.191638\t2.171117\t2.657034\t0.713141\t0.535862\t0.634274\n1666\t0.191113\t2.171032\t2.657788\t0.712245\t0.535781\t0.634274\n1667\t0.190785\t2.170947\t2.658543\t0.711349\t0.535701\t0.634274\n1668\t0.190617\t2.170862\t2.659297\t0.710454\t0.535621\t0.634232\n1669\t0.190448\t2.170777\t2.660052\t0.709558\t0.53554\t0.634157\n1670\t0.19028\t2.170692\t2.660806\t0.708663\t0.53546\t0.634082\n1671\t0.190112\t2.170607\t2.661561\t0.707767\t0.535379\t0.634007\n1672\t0.189943\t2.170522\t2.662315\t0.706872\t0.535299\t0.633933\n1673\t0.189775\t2.170437\t2.66307\t0.705976\t0.535218\t0.633858\n1674\t0.189607\t2.170352\t2.663824\t0.705081\t0.535138\t0.633783\n1675\t0.189438\t2.170267\t2.664579\t0.704185\t0.535057\t0.633708\n1676\t0.18927\t2.170182\t2.665333\t0.703289\t0.534977\t0.633633\n1677\t0.189102\t2.170097\t2.666088\t0.702394\t0.534896\t0.633559\n1678\t0.188933\t2.170039\t2.667384\t0.701498\t0.534816\t0.633484\n1679\t0.188765\t2.170018\t2.669403\t0.700603\t0.534735\t0.633409\n1680\t0.188597\t2.169996\t2.671422\t0.699707\t0.534655\t0.633334\n1681\t0.188428\t2.169975\t2.673441\t0.698812\t0.534574\t0.63326\n1682\t0.188316\t2.169954\t2.67546\t0.697916\t0.534494\t0.633185\n1683\t0.188367\t2.169933\t2.677479\t0.69702\t0.534413\t0.63311\n1684\t0.188418\t2.169911\t2.679498\t0.696125\t0.534333\t0.633035\n1685\t0.188469\t2.16989\t2.681517\t0.695229\t0.534281\t0.632961\n1686\t0.18852\t2.169869\t2.683536\t0.694334\t0.534281\t0.632886\n1687\t0.188571\t2.169848\t2.685555\t0.693438\t0.534281\t0.632811\n1688\t0.188622\t2.169826\t2.687574\t0.692749\t0.534281\t0.632736\n1689\t0.188673\t2.169805\t2.689593\t0.692749\t0.534281\t0.632662\n1690\t0.188724\t2.169784\t2.691612\t0.692749\t0.534281\t0.632587\n1691\t0.188775\t2.169763\t2.693631\t0.692749\t0.534281\t0.63252\n1692\t0.188826\t2.169741\t2.69565\t0.692749\t0.534281\t0.63252\n1693\t0.188877\t2.169658\t2.697778\t0.692749\t0.534281\t0.63252\n1694\t0.188928\t2.169158\t2.700628\t0.692749\t0.534281\t0.63252\n1695\t0.188979\t2.168659\t2.703478\t0.692749\t0.534281\t0.63252\n1696\t0.18903\t2.168159\t2.706327\t0.692749\t0.534281\t0.63252\n1697\t0.189081\t2.16766\t2.709177\t0.692749\t0.534281\t0.63252\n1698\t0.18944\t2.16716\t2.712027\t0.692749\t0.534281\t0.63252\n1699\t0.189813\t2.166661\t2.714877\t0.692749\t0.534281\t0.63252\n1700\t0.190185\t2.166162\t2.717727\t0.692749\t0.534281\t0.63252\n1701\t0.190558\t2.165662\t2.720577\t0.692749\t0.534281\t0.63252\n1702\t0.19093\t2.165163\t2.723427\t0.692749\t0.534281\t0.63252\n1703\t0.191302\t2.164663\t2.726276\t0.692749\t0.534281\t0.63252\n1704\t0.191675\t2.164164\t2.729126\t0.692749\t0.534281\t0.63252\n1705\t0.192047\t2.163664\t2.731976\t0.692749\t0.534281\t0.63252\n1706\t0.192419\t2.163165\t2.735387\t0.692749\t0.534281\t0.63252\n1707\t0.192792\t2.162665\t2.739908\t0.692749\t0.534281\t0.63252\n1708\t0.193164\t2.162166\t2.744429\t0.692749\t0.534281\t0.63252\n1709\t0.193537\t2.161339\t2.74895\t0.692749\t0.534281\t0.63252\n1710\t0.193909\t2.160447\t2.753471\t0.692749\t0.534281\t0.63252\n1711\t0.194281\t2.159554\t2.757992\t0.692749\t0.534281\t0.63252\n1712\t0.194654\t2.158661\t2.761471\t0.692749\t0.534281\t0.63252\n1713\t0.195265\t2.157769\t2.764277\t0.692749\t0.534281\t0.63252\n1714\t0.196\t2.156876\t2.767084\t0.692749\t0.534281\t0.63252\n1715\t0.196734\t2.155983\t2.76989\t0.692749\t0.534281\t0.63252\n1716\t0.197469\t2.155091\t2.772697\t0.692749\t0.534281\t0.63252\n1717\t0.198204\t2.154198\t2.775503\t0.692749\t0.534281\t0.63252\n1718\t0.198938\t2.153306\t2.77831\t0.692749\t0.534281\t0.63252\n1719\t0.199673\t2.152413\t2.781116\t0.692749\t0.534281\t0.63252\n1720\t0.200407\t2.15152\t2.783857\t0.692749\t0.534281\t0.63252\n1721\t0.201142\t2.150628\t2.786571\t0.692749\t0.534281\t0.63252\n1722\t0.201876\t2.149735\t2.789286\t0.692749\t0.534281\t0.63252\n1723\t0.202611\t2.148842\t2.792\t0.692749\t0.534281\t0.63252\n1724\t0.203345\t2.147731\t2.794714\t0.692749\t0.534281\t0.63252\n1725\t0.20408\t2.146428\t2.797428\t0.692749\t0.534281\t0.63252\n1726\t0.204815\t2.145126\t2.800142\t0.692749\t0.534281\t0.63252\n1727\t0.205549\t2.143823\t2.802856\t0.692749\t0.534281\t0.63252\n1728\t0.206515\t2.142521\t2.80557\t0.692749\t0.534281\t0.63252\n1729\t0.207887\t2.141218\t2.808285\t0.692749\t0.534281\t0.63252\n1730\t0.209258\t2.139916\t2.805334\t0.692749\t0.534281\t0.63252\n1731\t0.21063\t2.138613\t2.801655\t0.692749\t0.534281\t0.63252\n1732\t0.212002\t2.137311\t2.797975\t0.692749\t0.534281\t0.63252\n1733\t0.213374\t2.136008\t2.794296\t0.692749\t0.534281\t0.63252\n1734\t0.214746\t2.134706\t2.790617\t0.692749\t0.534281\t0.63252\n1735\t0.216118\t2.133403\t2.787527\t0.692749\t0.534281\t0.63252\n1736\t0.21749\t2.132101\t2.785288\t0.692749\t0.534281\t0.63252\n1737\t0.218862\t2.130798\t2.783049\t0.692749\t0.534281\t0.63252\n1738\t0.220234\t2.129496\t2.78081\t0.692749\t0.534281\t0.63252\n1739\t0.221606\t2.128068\t2.778572\t0.692749\t0.534281\t0.63252\n1740\t0.222977\t2.126235\t2.776333\t0.692749\t0.534281\t0.63252\n1741\t0.224297\t2.124403\t2.774094\t0.692749\t0.534281\t0.63252\n1742\t0.22532\t2.122571\t2.771855\t0.692749\t0.534281\t0.63252\n1743\t0.226344\t2.120739\t2.769616\t0.692749\t0.534281\t0.63252\n1744\t0.227367\t2.118906\t2.770863\t0.692749\t0.534281\t0.63252\n1745\t0.22839\t2.117074\t2.772247\t0.692749\t0.534281\t0.63252\n1746\t0.229414\t2.115242\t2.773631\t0.692749\t0.534281\t0.63252\n1747\t0.230437\t2.113409\t2.775014\t0.692749\t0.534281\t0.63252\n1748\t0.231461\t2.111577\t2.776398\t0.692749\t0.534281\t0.63252\n1749\t0.232484\t2.109745\t2.777782\t0.692749\t0.534281\t0.63252\n1750\t0.233507\t2.107912\t2.779323\t0.692749\t0.534281\t0.63252\n1751\t0.234531\t2.10608\t2.782125\t0.692749\t0.534281\t0.63252\n1752\t0.235554\t2.104248\t2.784927\t0.692749\t0.534281\t0.63252\n1753\t0.236911\t2.102415\t2.787728\t0.692749\t0.534281\t0.63252\n1754\t0.239434\t2.100583\t2.79053\t0.692749\t0.534281\t0.63252\n1755\t0.241957\t2.098252\t2.793331\t0.692749\t0.534281\t0.63252\n1756\t0.244481\t2.095888\t2.796133\t0.692749\t0.534281\t0.63252\n1757\t0.247004\t2.093524\t2.798877\t0.692749\t0.534281\t0.63252\n1758\t0.249527\t2.09116\t2.800164\t0.692749\t0.534281\t0.63252\n1759\t0.252051\t2.088796\t2.801451\t0.692749\t0.534281\t0.63252\n1760\t0.254574\t2.086432\t2.802737\t0.692749\t0.534281\t0.63252\n1761\t0.257097\t2.084068\t2.804024\t0.692749\t0.534281\t0.63252\n1762\t0.259621\t2.081704\t2.805311\t0.692749\t0.534281\t0.63252\n1763\t0.262144\t2.07934\t2.806598\t0.692749\t0.534281\t0.63252\n1764\t0.263948\t2.076976\t2.807885\t0.692749\t0.534281\t0.63252\n1765\t0.26567\t2.074612\t2.809172\t0.692749\t0.534281\t0.63252\n1766\t0.267393\t2.072248\t2.809266\t0.692749\t0.534281\t0.63252\n1767\t0.269115\t2.069884\t2.809085\t0.692749\t0.534281\t0.63252\n1768\t0.270838\t2.065842\t2.808904\t0.692749\t0.534281\t0.63252\n1769\t0.272561\t2.061168\t2.808724\t0.692749\t0.534281\t0.63252\n1770\t0.274283\t2.056495\t2.808543\t0.692749\t0.534281\t0.63252\n1771\t0.276006\t2.051822\t2.808363\t0.692749\t0.534281\t0.63252\n1772\t0.277729\t2.047148\t2.808182\t0.692749\t0.534281\t0.63252\n1773\t0.279451\t2.042475\t2.808001\t0.692749\t0.534281\t0.63252\n1774\t0.281174\t2.037801\t2.807821\t0.692749\t0.534281\t0.63252\n1775\t0.282828\t2.033128\t2.80764\t0.692749\t0.534281\t0.63252\n1776\t0.283667\t2.028455\t2.807459\t0.692749\t0.534281\t0.63252\n1777\t0.284506\t2.024356\t2.807279\t0.692749\t0.534281\t0.63252\n1778\t0.285345\t2.020519\t2.807098\t0.692749\t0.534281\t0.63252\n1779\t0.286185\t2.016682\t2.806917\t0.692749\t0.534281\t0.63252\n1780\t0.287024\t2.012845\t2.806737\t0.692749\t0.534281\t0.63252\n1781\t0.287863\t2.009008\t2.80658\t0.692749\t0.534281\t0.63252\n1782\t0.288702\t2.005171\t2.806445\t0.692749\t0.534281\t0.63252\n1783\t0.289541\t2.001334\t2.80631\t0.692749\t0.534281\t0.63252\n1784\t0.29038\t1.997497\t2.806176\t0.692749\t0.534281\t0.63252\n1785\t0.29122\t1.99366\t2.806041\t0.692749\t0.534281\t0.63252\n1786\t0.292059\t1.99149\t2.805906\t0.692749\t0.534281\t0.63252\n1787\t0.292898\t1.989454\t2.805771\t0.692749\t0.534281\t0.63252\n1788\t0.293737\t1.987419\t2.805637\t0.692749\t0.534281\t0.63252\n1789\t0.29445\t1.985384\t2.805502\t0.692749\t0.534281\t0.63252\n1790\t0.294547\t1.983348\t2.805367\t0.692749\t0.534281\t0.63252\n1791\t0.294645\t1.981313\t2.805233\t0.692749\t0.534281\t0.63252\n1792\t0.294742\t1.979278\t2.805098\t0.692749\t0.534281\t0.63252\n1793\t0.294839\t1.977242\t2.804963\t0.692749\t0.534281\t0.63252\n1794\t0.294936\t1.975207\t2.804829\t0.692749\t0.534281\t0.63252\n1795\t0.295034\t1.973172\t2.804694\t0.692749\t0.534281\t0.63252\n1796\t0.295131\t1.971136\t2.804682\t0.692749\t0.534281\t0.63252\n1797\t0.295228\t1.969101\t2.804682\t0.692749\t0.534281\t0.63252\n1798\t0.295325\t1.968747\t2.804682\t0.692749\t0.534281\t0.63252\n"
  # "S"
  # "A"
  n1 = property on="Array 2" class="Arr (strict)"() -> ("Index Values"=w54:u32[])  [unwired: 2 in, 2 out]
  n2 = Index Array(array=w54) -> (element #1=w52:u32, element #2=w51:u32)  [unwired: 2 in]
  n3 = Index Array(array="Array 2", index (row)=w52, index (col)=w51) -> (element=w50:T4)
  n4 = Build Array(w61, w62) -> (w60:string[])
  n5 = for {
    tunnel: w60 -> [w78] mode=indexing
    tunnel: [w82] -> w59 mode=indexing
    tunnel: [w81] -> w58 mode=indexing
    tunnel: [w79] -> w57 mode=indexing
    n6 = Spreadsheet String To Array(format string="", spreadsheet string=w78) -> (array=w84:dbl[][])  [unwired: 2 in]
    n7 = Index Array(array=w84, index (col) #1=0 ("disabled index (col)"), index (col) #2=1 ("index (col)"), index (col) #3=2 ("index (col)")) -> (element #1=w80:dbl[], element #2=w76:dbl[], element #3=w75:dbl[])  [unwired: 3 in]
    n8 = expression code="x/(100*exp(1))"(w75) -> (w74:dbl[])
    n9 = expression code="x/(100*exp(1))"(w76) -> (w73:dbl[])
    n10 = Array Max & Min(array=w80) -> (max value=w82:dbl, min value=w81:dbl)  [unwired: 2 out]
    n11 = Bundle(w80, w73, w74) -> (w79:cluster{dbl[], dbl[], dbl[]})  [unwired: 1 in]
  }
  n12 = Unbundle(w50) -> ("Slab C=A, T=S 2"=w27:T5, "Supra-Space Mini Map"=w49:cluster{dbl[], dbl[]}[])  [unwired: 2 out]
  n13 = Index Array(array=w49, index=0) -> (element=w47:cluster{dbl[], dbl[]})
  n14 = for {
    tunnel: w27 -> [w93] mode=indexing
    tunnel: [w91] -> w30
    tunnel: [w90] -> w45 mode=indexing
    tunnel: [w89] -> w28 mode=indexing
    tunnel: [w88] -> w29
    n15 = Unbundle(w93) -> ("Color and Time Graph"=w92:cluster{dbl[], dbl[]}[], "String"=w86:string)  [unwired: 1 out]
    n16 = Match Pattern(string=w86, regular expression="=") -> (after substring=w85:string)  [unwired: 1 in, 3 out]
    n17 = Fract/Exp String To Number(string=w85) -> (number=w89:dbl)  [unwired: 3 in, 1 out]
    n18 = for {
      tunnel: w92 -> [w99] mode=indexing
      tunnel: [w98] -> w91
      tunnel: [w97] -> w90 mode=indexing
      tunnel: [w95] -> w88 mode=indexing
      i -> [w96]
      n19 = Unbundle(w99) -> (w98:dbl[], w97:dbl[])
      n20 = property on="Color and Time Graph" class="XYGraph (strict)"("Active Plot"=w96) -> ("Plot.Plot Name"=w94:string)  [unwired: 2 in, 2 out]
      n21 = Fract/Exp String To Number(string=w94) -> (number=w95:dbl)  [unwired: 3 in, 1 out]
    }
  }
  "Values" <- w45
  "Vector - Depth" <- w30
  "Vector - Scattering" <- w29
  "Vector - Abs" <- w28
  n22 = Unbundle(w47) -> (w46:dbl[])  [unwired: 1 out]
  n23 = Index Array(array=w46) -> (element=w43:dbl)  [unwired: 1 in]
  "WD" <- w43
  n24 = Divide(x=w43, y=w40) -> (x/y=w42:dbl)
  n25 = Increment(x=w42) -> (x+1=w41:dbl)
  n26 = for {
    N: w41 -> [_]
    tunnel: w40 -> [w101]
    tunnel: [w100] -> w25 mode=indexing
    i -> [w102]
    n27 = Multiply(x=w101, y=w102) -> (x*y=w100:dbl)
  }
  "New Vector - Depth" <- w25
  n28 = Array Max & Min(array=w59) -> ()  [unwired: 4 out]
  n29 = Array Max & Min(array=w58) -> ()  [unwired: 4 out]
  n30 = Bundle(w30, w29, w28) -> (w44:cluster{dbl[], dbl[], dbl[]})  [unwired: 1 in]
  "Axis Vectors" <- w44
  n31 = Subtract(x=w24, y=w31) -> (x-y=w69:dbl)
  n32 = Divide(x=w69, y=w66) -> (x/y=w68:dbl)
  n33 = Round Toward -Infinity(1:w68) -> (0:w67:dbl)
  n34 = call <vilib>:"Color to RGB.vi"("Color"="Color 2") -> ("R"=w32:u8, "G"=w33:u8, "B"=w34:u8)  [unwired: 1 out]
  n35 = call <vilib>:"Color to RGB.vi"("Color"="Color 1") -> ("R"=w35:u8, "G"=w36:u8, "B"=w37:u8)  [unwired: 1 out]
  n36 = Increment(x=w67) -> (x+1=w23:dbl)
  n37 = for {
    N: w23 -> [_]
    tunnel: w31 -> [w104]
    tunnel: w66 -> [w107]
    tunnel: [w103] -> w26 mode=indexing
    i -> [w106]
    n38 = Multiply(x=w107, y=w106) -> (x*y=w105:dbl)
    n39 = Add(x=w104, y=w105) -> (x+y=w103:dbl)
  }
  "Vector - Wavelength" <- w26
  n40 = Spreadsheet String To Array(format string="", spreadsheet string=w6) -> (array=w5:dbl[][])  [unwired: 2 in]
  n41 = Index Array(array=w5, index (col) #1=0 ("disabled index (col)")) -> (element #1=w3:dbl[], element #2=w2:dbl[])  [unwired: 3 in]
  n42 = expression code="x/(100*exp(1))"(w2) -> (w1:dbl[])
  n43 = for {
    tunnel: w26 -> [w115] mode=indexing
    tunnel: [w112] -> w55 mode=indexing
    tunnel: w57 -> [w113]
    tunnel: [w110] -> w56 mode=indexing
    tunnel: w3 -> [w109]
    tunnel: w1 -> [w108]
    n44 = for {
      tunnel: w115 -> [w120]
      tunnel: [w116] -> w114 mode=indexing if=w122
      tunnel: w113 -> [w128] mode=indexing
      tunnel: [w117] -> w111 mode=indexing if=w122
      tunnel: w109 -> [w121]
      tunnel: w108 -> [w118]
      n45 = Unbundle(w128) -> (w125:dbl[], w127:dbl[], w126:dbl[])
      n46 = Array Max & Min(array=w125) -> (max value=w124:dbl, min value=w123:dbl)  [unwired: 2 out]
      n47 = Threshold 1D Array(2:w120, 3:w125) -> (0:w129:dbl)  [unwired: 1 in]
      n48 = Threshold 1D Array(2:w120, 3:w121) -> (0:w119:dbl)  [unwired: 1 in]
      n49 = In Range and Coerce(upper limit=w124, x=w120, lower limit=w123) -> (In Range?=w122:bool)  [unwired: 1 out]
      n50 = Interpolate 1D Array(1:w129, 2:w127) -> ()  [unwired: 1 out]
      n51 = Interpolate 1D Array(1:w129, 2:w126) -> (0:w117:dbl)
      n52 = Interpolate 1D Array(1:w119, 2:w118) -> (0:w116:dbl)
    }
    n53 = call-poly <vilib>:"Mean.vi"("X"=w114) -> ("mean"=w112:dbl)  [unwired: 1 out]
    n54 = call-poly <vilib>:"Mean.vi"("X"=w111) -> ("mean"=w110:dbl)  [unwired: 1 out]
  }
  n55 = call <vilib>:"Color to RGB.vi"("Color"="Color 3") -> ("R"=w18:u8, "G"=w17:u8, "B"=w16:u8)  [unwired: 1 out]
  n56 = call <vilib>:"Color to RGB.vi"("Color"="Color 2") -> ("R"=w15:u8, "G"=w14:u8, "B"=w13:u8)  [unwired: 1 out]
  n57 = for {
    tunnel: w26 -> [w134] mode=indexing
    tunnel: w56 -> [w137] mode=indexing
    tunnel: w55 -> [w136] mode=indexing
    tunnel: w25 -> [w135]
    tunnel: [w130] -> w39 mode=indexing
    n58 = for {
      tunnel: w137 -> [w138]
      tunnel: w136 -> [w139]
      tunnel: [w141] -> w131 mode=indexing
      tunnel: w135 -> [w140] mode=indexing
      n59 = Bundle(w140, "mean"=w138, "mean"=w139) -> (w141:cluster{dbl, "mean":dbl, "mean":dbl})  [unwired: 1 in]
    }
    n60 = Format Into String(format string="%#f nm", w134) -> (resulting string=w132:string)  [unwired: 2 in, 1 out]
    n61 = Bundle(w132, w131) -> (w130:T6)  [unwired: 1 in]
  }
  "Graphs" <- w39
  n62 = for {
    N -> [w146]
    tunnel: w44 -> [w152]
    tunnel: w45 -> [w151]
    tunnel: w39 -> [w150] mode=indexing
    tunnel: [w147] -> w70 mode=indexing
    tunnel: [w142] -> w22 mode=indexing
    i -> [w145]
    n63 = Unbundle(w150) -> (w142:string, w144:cluster{dbl, "mean":dbl, "mean":dbl}[])
    n64 = for {
      tunnel: w152 -> [w157]
      tunnel: [w156] -> w148 mode=indexing
      tunnel: w151 -> [w155]
      tunnel: w144 -> [w154] mode=indexing
      tunnel: [w153] -> w149 mode=indexing
      n65 = call "Trilinear - Interpolation.vi"("XYZ Point"=w154, "Axis Vectors"=w157, "Values"=w155) -> ("Interpolated Value"=w156:dbl)  [unwired: 7 in, 1 out]
      n66 = Unbundle(w154) -> (w153:dbl)  [unwired: 2 out]
    }
    n67 = property on="Effects by Wavelength" class="XYGraph (strict)"("LegNumRows"=w146, "Active Plot"=w145, "Plot.Plot Name"=w142, "Plot.Point Style"=u8 0) -> ()  [unwired: 2 in, 2 out]
    n68 = Bundle(w149, w148) -> (w147:cluster{dbl[], dbl[]})  [unwired: 1 in]
  }
  "Effects by Wavelength" <- w70
  n69 = Array Size(array=w22) -> (size(s)=w21:i32)
  n70 = expression code="x/2"(w21) -> (w20:i32)
  n71 = Split 1D Array(array=w22, index=w20) -> (first subarray=w19:string[], second subarray=w10:string[])
  n72 = for {
    N -> [w159]
    tunnel: w32 -> [w180]
    tunnel: w33 -> [w179]
    tunnel: w34 -> [w178]
    tunnel: w35 -> [w177]
    tunnel: w36 -> [w176]
    tunnel: w37 -> [w175]
    tunnel: w19 -> [w162] mode=indexing
    tunnel: [w159] -> w9
    tunnel: [w158] -> w8
    i -> [w182]
    n73 = Decrement(x=w159) -> (x-1=w181:i32)
    n74 = Max & Min(x=w181, y=1) -> (max(x,y)=w161:i32)  [unwired: 1 out]
    n75 = Divide(x=w182, y=w161) -> (x/y=w174:dbl)
    n76 = Multiply(x=w174, y=w180) -> (x*y=w168:dbl)
    n77 = Multiply(x=w174, y=w179) -> (x*y=w169:dbl)
    n78 = Multiply(x=w174, y=w178) -> (x*y=w172:dbl)
    n79 = expression code="1-x"(w174) -> (w164:dbl)
    n80 = Multiply(x=w164, y=w177) -> (x*y=w170:dbl)
    n81 = Multiply(x=w164, y=w176) -> (x*y=w171:dbl)
    n82 = Multiply(x=w164, y=w175) -> (x*y=w173:dbl)
    n83 = Add(x=w168, y=w170) -> (x+y=w167:dbl)
    n84 = Add(x=w172, y=w173) -> (x+y=w165:dbl)
    n85 = Add(x=w169, y=w171) -> (x+y=w166:dbl)
    n86 = call <vilib>:"RGB to Color.vi"("B"=w165, "G"=w166, "R"=w167) -> ("Color"=w163:u32)
    n87 = property on="Effects by Wavelength" class="XYGraph (strict)"("Active Plot"=w182, "Plot.Point Style"=u8 0, "Plot.Plot Color"=w163, "Plot.Fill/Pt. Color"=w163, "Plot.Plot Name"=w162) -> (error out=w158:errorcluster)  [unwired: 2 in, 1 out]
  }
  n88 = for {
    N -> [w186]
    tunnel: w18 -> [w210]
    tunnel: w17 -> [w209]
    tunnel: w16 -> [w208]
    tunnel: w15 -> [w207]
    tunnel: w14 -> [w206]
    tunnel: w13 -> [w205]
    tunnel: w10 -> [w192] mode=indexing
    tunnel: w9 -> [w187]
    tunnel: w8 -> [w189]
    i -> [w212]
    n89 = Decrement(x=w186) -> (x-1=w211:i32)
    n90 = Max & Min(x=w211, y=1) -> (max(x,y)=w191:i32)  [unwired: 1 out]
    n91 = Divide(x=w212, y=w191) -> (x/y=w204:dbl)
    n92 = Multiply(x=w204, y=w210) -> (x*y=w198:dbl)
    n93 = Multiply(x=w204, y=w209) -> (x*y=w199:dbl)
    n94 = Multiply(x=w204, y=w208) -> (x*y=w202:dbl)
    n95 = expression code="1-x"(w204) -> (w194:dbl)
    n96 = Multiply(x=w194, y=w207) -> (x*y=w200:dbl)
    n97 = Multiply(x=w194, y=w206) -> (x*y=w201:dbl)
    n98 = Multiply(x=w194, y=w205) -> (x*y=w203:dbl)
    n99 = Add(x=w187, y=w212) -> (x+y=w188:i32)
    n100 = Add(x=w198, y=w200) -> (x+y=w197:dbl)
    n101 = Add(x=w187, y=w186) -> (x+y=w185:i32)
    n102 = Add(x=w202, y=w203) -> (x+y=w195:dbl)
    n103 = Add(x=w199, y=w201) -> (x+y=w196:dbl)
    n104 = call <vilib>:"RGB to Color.vi"("B"=w195, "G"=w196, "R"=w197) -> ("Color"=w193:u32)
    n105 = property on="Effects by Wavelength" class="XYGraph (strict)"(error in=w189, "Active Plot"=w188, "Plot.Point Style"=u8 0, "Plot.Plot Color"=w193, "Plot.Fill/Pt. Color"=w193, "Plot.Plot Name"=w192, "LegNumRows"=w185, "Plot.Line Width"=u8 2) -> ()  [unwired: 1 in, 2 out]
  }
  n106 = Bundle(w26, w55) -> (w65:cluster{dbl[], dbl[]})  [unwired: 1 in]
  n107 = Bundle(w26, w56) -> (w64:cluster{dbl[], dbl[]})  [unwired: 1 in]
  n108 = Build Array(w65, w64) -> (→"Effects by Wavelength 2":cluster{dbl[], dbl[]}[])
